vi "Main.vi"() -> ()   [LabVIEW 2019]
uses:
  Code/typeDefs/Parameters.ctl
  Code/typeDefs/MFCIn.ctl
  Code/typeDefs/MFCOut.ctl
  Code/typeDefs/keithleySettings.ctl
  Code/typeDefs/MFCSet.ctl
  <vilib>/Utility/miscctls.llb/LVPointTypeDef.ctl
  <vilib>/DAQmx/read.llb/DAQmx Read (Analog 1D Wfm NChan NSamp).vi
  <vilib>/Analysis/baseanly.llb/Mean (DBL).vi
  <vilib>/DAQmx/write.llb/DAQmx Write (Digital 1D Bool NChan 1Samp 1Line).vi
  <vilib>/DAQmx/write.llb/DAQmx Write (Analog DBL 1Chan 1Samp).vi
  <vilib>/DAQmx/create/channels.llb/DAQmx Create Channel (AO-Voltage-Basic).vi
  <vilib>/DAQmx/miscellaneous.llb/DAQmx Fill In Error Info.vi
  <vilib>/DAQmx/create/channels.llb/DAQmx Create Channel (DO-Digital Output).vi
  <vilib>/DAQmx/create/channels.llb/DAQmx Create Channel (AI-Voltage-Basic).vi
  <vilib>/DAQmx/configure/timing.llb/DAQmx Timing (Sample Clock).vi
  <vilib>/Instr/_visa.llb/VISA Configure Serial Port (Instr).vi
  Code/Scripts/Scripts.lvclass
  Code/SMU/SMU.lvclass
  Code/MFC/MFC.lvclass
  Code/DAQ/DAQ.lvclass
  <resource>/objmgr/daqmx.rc
  <vilib>/Analysis/NI_AALBase.lvlib
  Code/2231A/2231A.lvclass
  <instrlib>/Keithley DMM6500 DAQ6500 Series/Keithley DMM6500 DAQ6500 Series.lvlib
panel:
  out "Visible Resistance":dbl[](array[numeric]) caption="Resistance (Ohms)"
  in  "Names default":string[](array[string])=["Ethanol (%)", "RH (%)", "Temp (C)", "MFC A", "MFC B", "Resistance 1"]
  out "t0 2":dbl
  in  "DevBackgate":bool
  out "Read Time":dbl caption="Read Time (s)"
  out "t0":timestamp
  out "CvsV":T1(graph) caption="Current vs Voltage"
  in  "Timeout Stop":bool
  out "MFC Index":i32
  out "Names":string[](array[string])=["Ethanol (%)", "RH (%)", "Temp (C)", "MFC A", "MFC B", "Resistance 1"]
  in  "Stop":bool
  in  "Tab Control":T2(tab)=enum."Experiment"
  in  "AO_LED":tag="Dev1/ao0"
  in  "DO_Valves":tag="Dev1/port0/line0:1"
  in  "DAQ channels":tag="Dev1/ai0:2"
  in  "Keithley 2450 Sense":refnum<visa-resource-name>="GPIB0::1::INSTR"
  in  "MFC Config":T3={"Tare absP"=FALSE, "Tare Flow"=FALSE, "baud rate (9600)"=19200, "MFC COM Port"="COM5", "Device ID's"=["A", "B"]}
  in  "DAQ Config":T4={"RH/T Sensor VSS (V)"=5.048, "K0"=0.9054, "K1"=-2.995, "Offset"=0.0, "Gain"=1.0, "Samples/Channel/s"=1000.0, "Samples to Average"=1000.0} {"Offset" step=0.01 format="%_3f"; "K1" format="%#_13g"; "K0" format="%#_13g"; "RH/T Sensor VSS (V)" format="%.3g"}
  out "Unprocessed Samples in Queue":u32=5
  out "DPS":dbl=100.0 caption="Data Points / Second"
  in  "Keithley Config":T5={"Source Compliance (A)"=0.1, "Min Voltage (V)"=0.1, "Max Voltage (V)"=3.0, "Source Mode"=0, "Number of Points"=10} {"Number of Points" min=2 step=1; "Source Mode" items=["Voltage", "Current"]; "Min Voltage (V)" min=0.1}
  in  "Keithley wait":sgl caption="Read Delay (s)" min=0 max=100 step=0.25
  in  "DAQ 6510 Switch":refnum<visa-resource-name>="DAQ_6510"
  in  "# of Sensors":dbl=1.0 min=1.0 max=9.0 step=1.0
  in  "Keithley 2450 Source":refnum<visa-resource-name>="GPIB0::2::INSTR"
  in  "Duty Cycle":dbl=0.5 min=0.01 max=0.99 step=0.01
  in  "Freq":dbl=1.0 caption="Freq (Hz)" min=0.1 max=100.0 step=1.0
  in  "Strobe":bool
  in  "Hours to Run":dbl=24.0 min=0.02 max=100.0 step=0.25 format="%#_5g"
  in  "Aquire data":bool
  out "Start Time":timestamp format="%<%I:%M:%S %p>T"
  in  "MFC Set":T6[](array[typedef])=[{"MFC Set"=[{"String"="A", "MFC set"=1000.0}, {"String"="B", "MFC set"=25.0}], "set 1"=FALSE}, {"MFC Set"=[{"String"="A", "MFC set"=1000.0}, {"String"="B", "MFC set"=25.0}], "set 1"=TRUE}] {"MFC Set"."MFC set" step=10.0 format="%.2f"}
  in  "Voltage (V)":dbl(slide) min=0.0 max=10.0 step=0.1 scale=0.0..10.0
  in  "Valves":bool[](array[boolean])=[FALSE, FALSE]
  in  "Plot Data":bool
  out "End Time":timestamp format="%<%I:%M:%S %p>T"
  in  "Save to File":bool
  in  "File Name":string
  out "Current Time (s)":u32
  in  "Aquire data 2":bool
  in  "Test Script":u16(ring) items=["Backgate Test", "Example1", "Example1_rr_bg_40_Nat", "Jaewoo_Test - Copy", "None"]
  out "Script Contents":i32(listbox)
  in  "Sensors":bool[](array[boolean])=[TRUE, FALSE, FALSE, FALSE, FALSE, FALSE, FALSE, FALSE, FALSE]
  out "Backgate Display":cluster{"all rows":dbl[], "all rows":dbl[]}(graph)
  in  "Increment (V)":dbl=1.0 min=0.0 max=63.0
  in  "Range (V)":dbl=60.0 min=1.0 max=60.0
  in  "Backgate":bool
  in  "Style":u16(ring) items=["Ramp+-", "Pos-Neg", "Ramp", "0 Ramp", "Double+-"]
  out "BG Time (s)":dbl
  out "Computer Read Time (s)":dbl
  out "Keithley 2450 Source":errorcluster
  out "LED_AO":errorcluster
  out "3-Valve_DO":errorcluster
  out "DAQ_IO (RH,Temp,Eth)":errorcluster
  out "MFC_IO":errorcluster
  out "Keithley 2450 Sense":errorcluster
  out "DAQ 6510 Switch":errorcluster
  out "Resistance Proper":dbl[][](array[numeric]) caption="Resistance"
  in  "Clear DAQ":bool
  out "MFCArray":T7[](array[typedef])=[{"Gas"="", "Setpoint"=0.0, "MassFlow"=0.0, "T ºC"=0.0, "P(PSI)"=0.0, "ID"="-"}, {"Gas"="", "Setpoint"=0.0, "MassFlow"=0.0, "T ºC"=0.0, "P(PSI)"=0.0, "ID"="-"}] {"MassFlow" format="%.2f"; "Setpoint" format="%.2f"}
  out "Waveform Chart":waveform(dbl)[](graph)=[{"t0"=timestamp(3675342615.977705 s since 1904-01-01), "dt"=0.01, "Y"=[0.0007680409200236937]}, {"t0"=timestamp(3675342615.977705 s since 1904-01-01), "dt"=0.01, "Y"=[0.0105205510693704]}, {"t0"=timestamp(3675342615.977705 s since 1904-01-01), "dt"=0.01, "Y"=[89.00820200660893]}, {"t0"=timestamp(3675342615.977705 s since 1904-01-01), "dt"=0.01, "Y"=[117.62674839380017]}, {"t0"=timestamp(3675342615.977705 s since 1904-01-01), "dt"=0.01, "Y"=[0.0]}, {"t0"=timestamp(3675342615.977705 s since 1904-01-01), "dt"=0.01, "Y"=[0.0]}]
  out "T":dbl caption="T  (ºC)" format="%.2g"
  out "RH":dbl caption="RH  (%)" format="%.2g"
  out "Eth":dbl caption="Ethanol (%)" format="%.3g"
  # "Created By Lukas Scarfe\nEngineering Physics"
  # "Save to File"
  # "LED"
  # "1"
  # "2"
  # "Backgate Configuration"
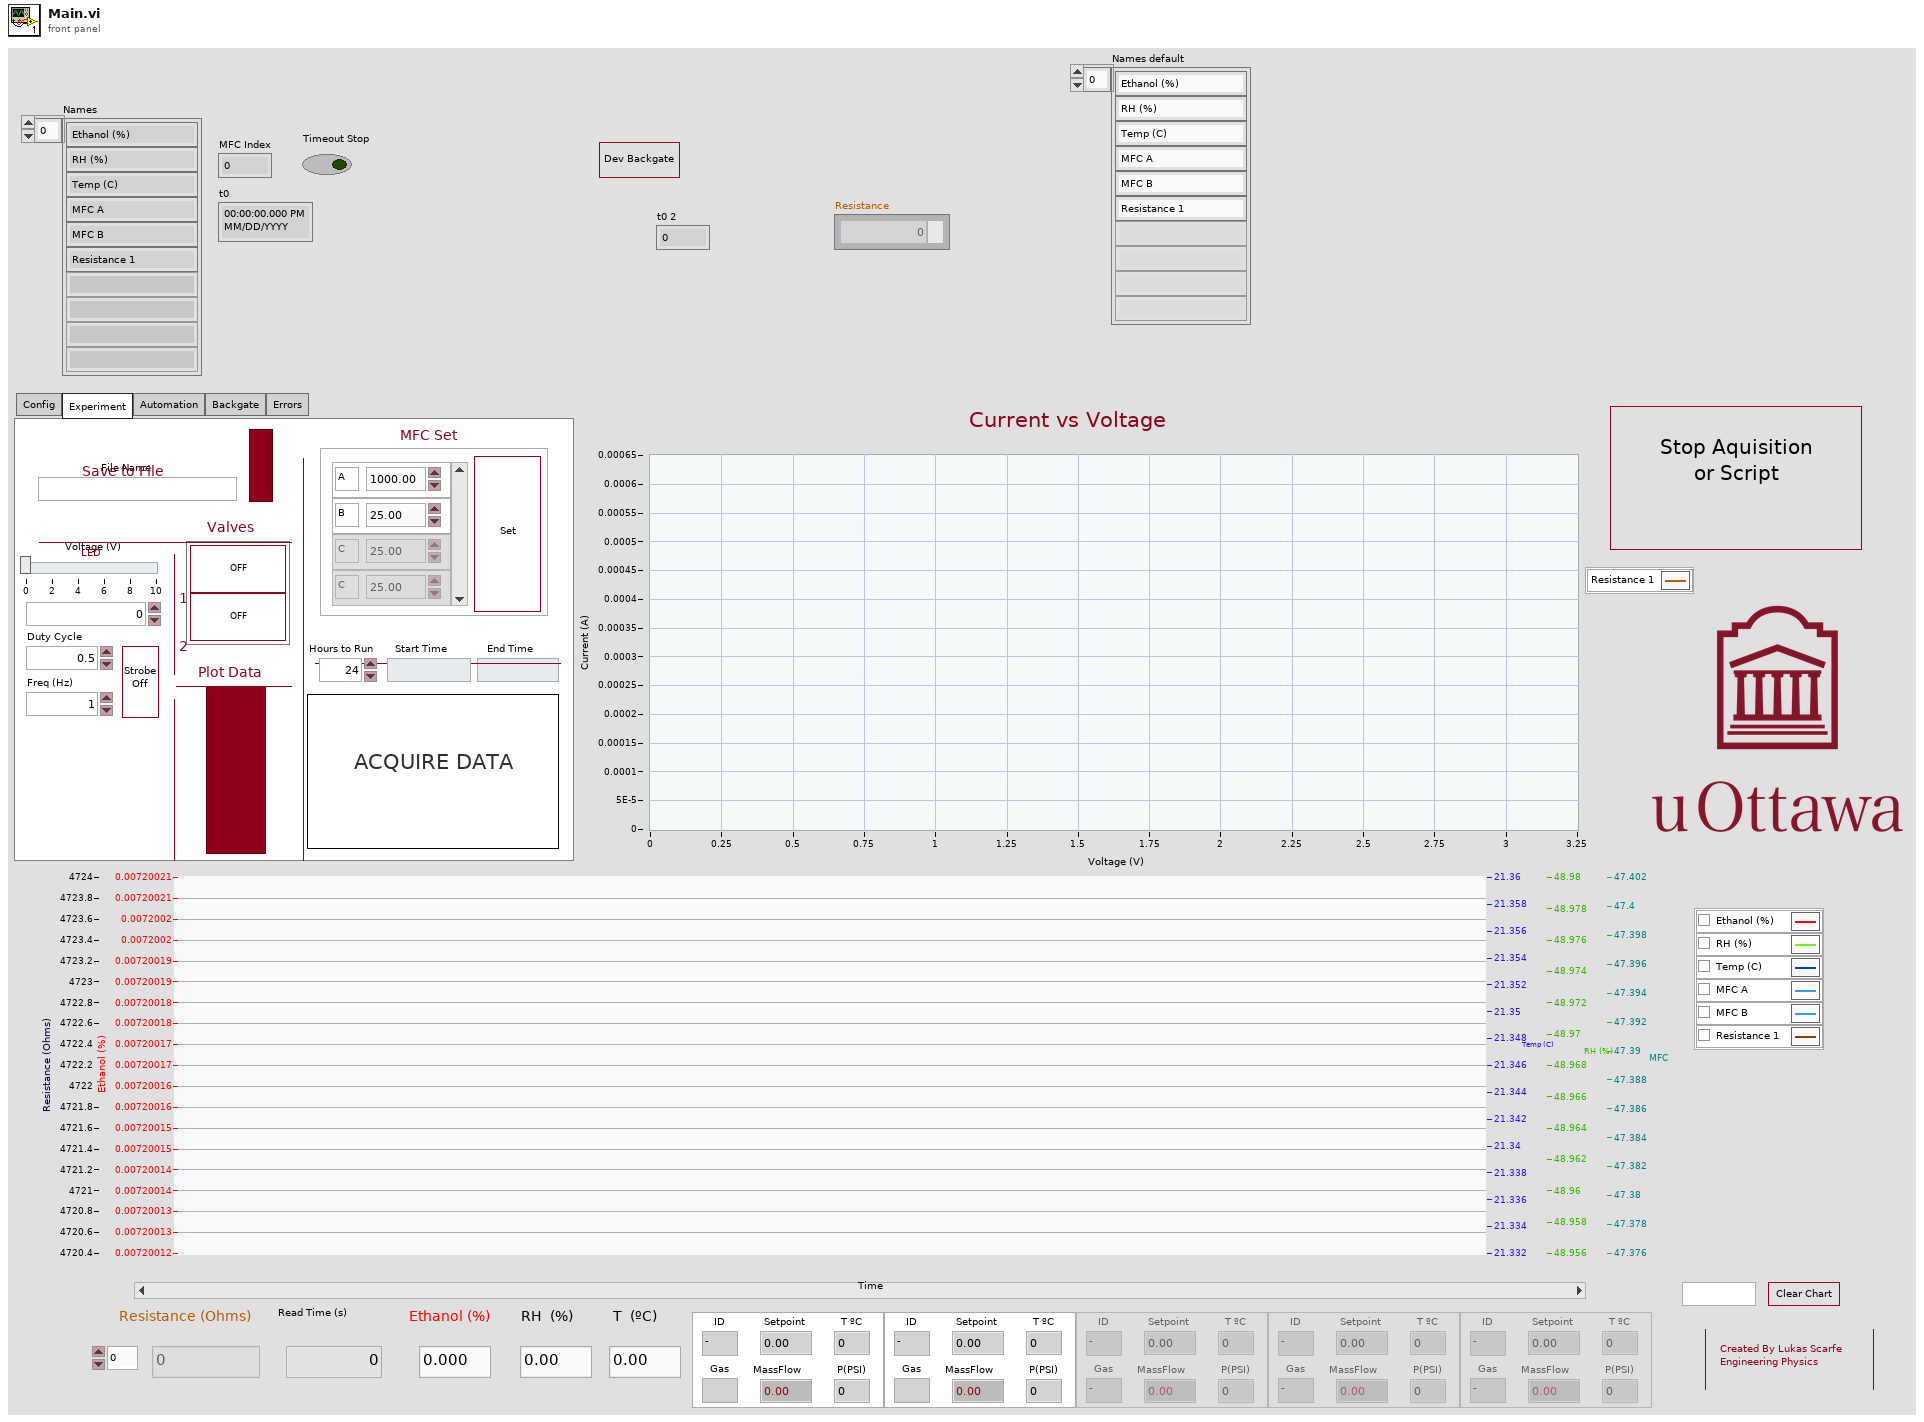
[diagram p1: front panel]
types:
  T1 = cluster{"All Values Out":sgl[], "All Values Out":sgl[]}[]
  T2 = enum32{"Config", "Experiment", "Automation", "Backgate", "Errors"}
  T3 = typedef "MFCIn.ctl" = cluster{"Tare absP":bool, "Tare Flow":bool, "baud rate (9600)":u32, "MFC COM Port":refnum<visa-resource-name>, "Device ID's":string[]}
  T4 = typedef "Parameters.ctl" = cluster{"RH/T Sensor VSS (V)":dbl, "K0":dbl, "K1":dbl, "Offset":dbl, "Gain":dbl, "Samples/Channel/s":dbl, "Samples to Average":dbl}
  T5 = typedef "keithleySettings.ctl" = cluster{"Source Compliance (A)":dbl, "Min Voltage (V)":dbl, "Max Voltage (V)":dbl, "Source Mode":u16, "Number of Points":u32}
  T6 = typedef "MFCSet.ctl" = cluster{"MFC Set":cluster{"String":string, "MFC set":dbl}[], "set 1":bool}
  T7 = typedef "MFCOut.ctl" = cluster{"Gas":string, "Setpoint":dbl, "MassFlow":dbl, "T ºC":dbl, "P(PSI)":dbl, "ID":string}
  T8 = enum32{"invalid app kind", "Development System", "Run Time System", "Student Edition", "Embedded LabVIEW", "Evaluation", "Custom"}
  T9 = typedef "LVPointTypeDef.ctl" = cluster{"Horizontal":i16, "Vertical":i16}
  T10 = cluster{"array":sgl[], "Best Linear Fit":dbl[]}[]
  T11 = enum8{"Enabled", "Disabled", "Disabled and Grayed Out"}
  T12 = cluster{"All Values Out":sgl[], "All Values Out":sgl[]}
  T13 = cluster{"MFC Set":cluster{"String":bool, "MFC set":bool}[], "set 1":bool}
  T14 = typedef "Graph.ctl" = cluster{"Ethanol":dbl, "RH":dbl, "Temp":dbl, "MFC A":dbl, "MFC B":dbl, "Resistances":dbl[][]}
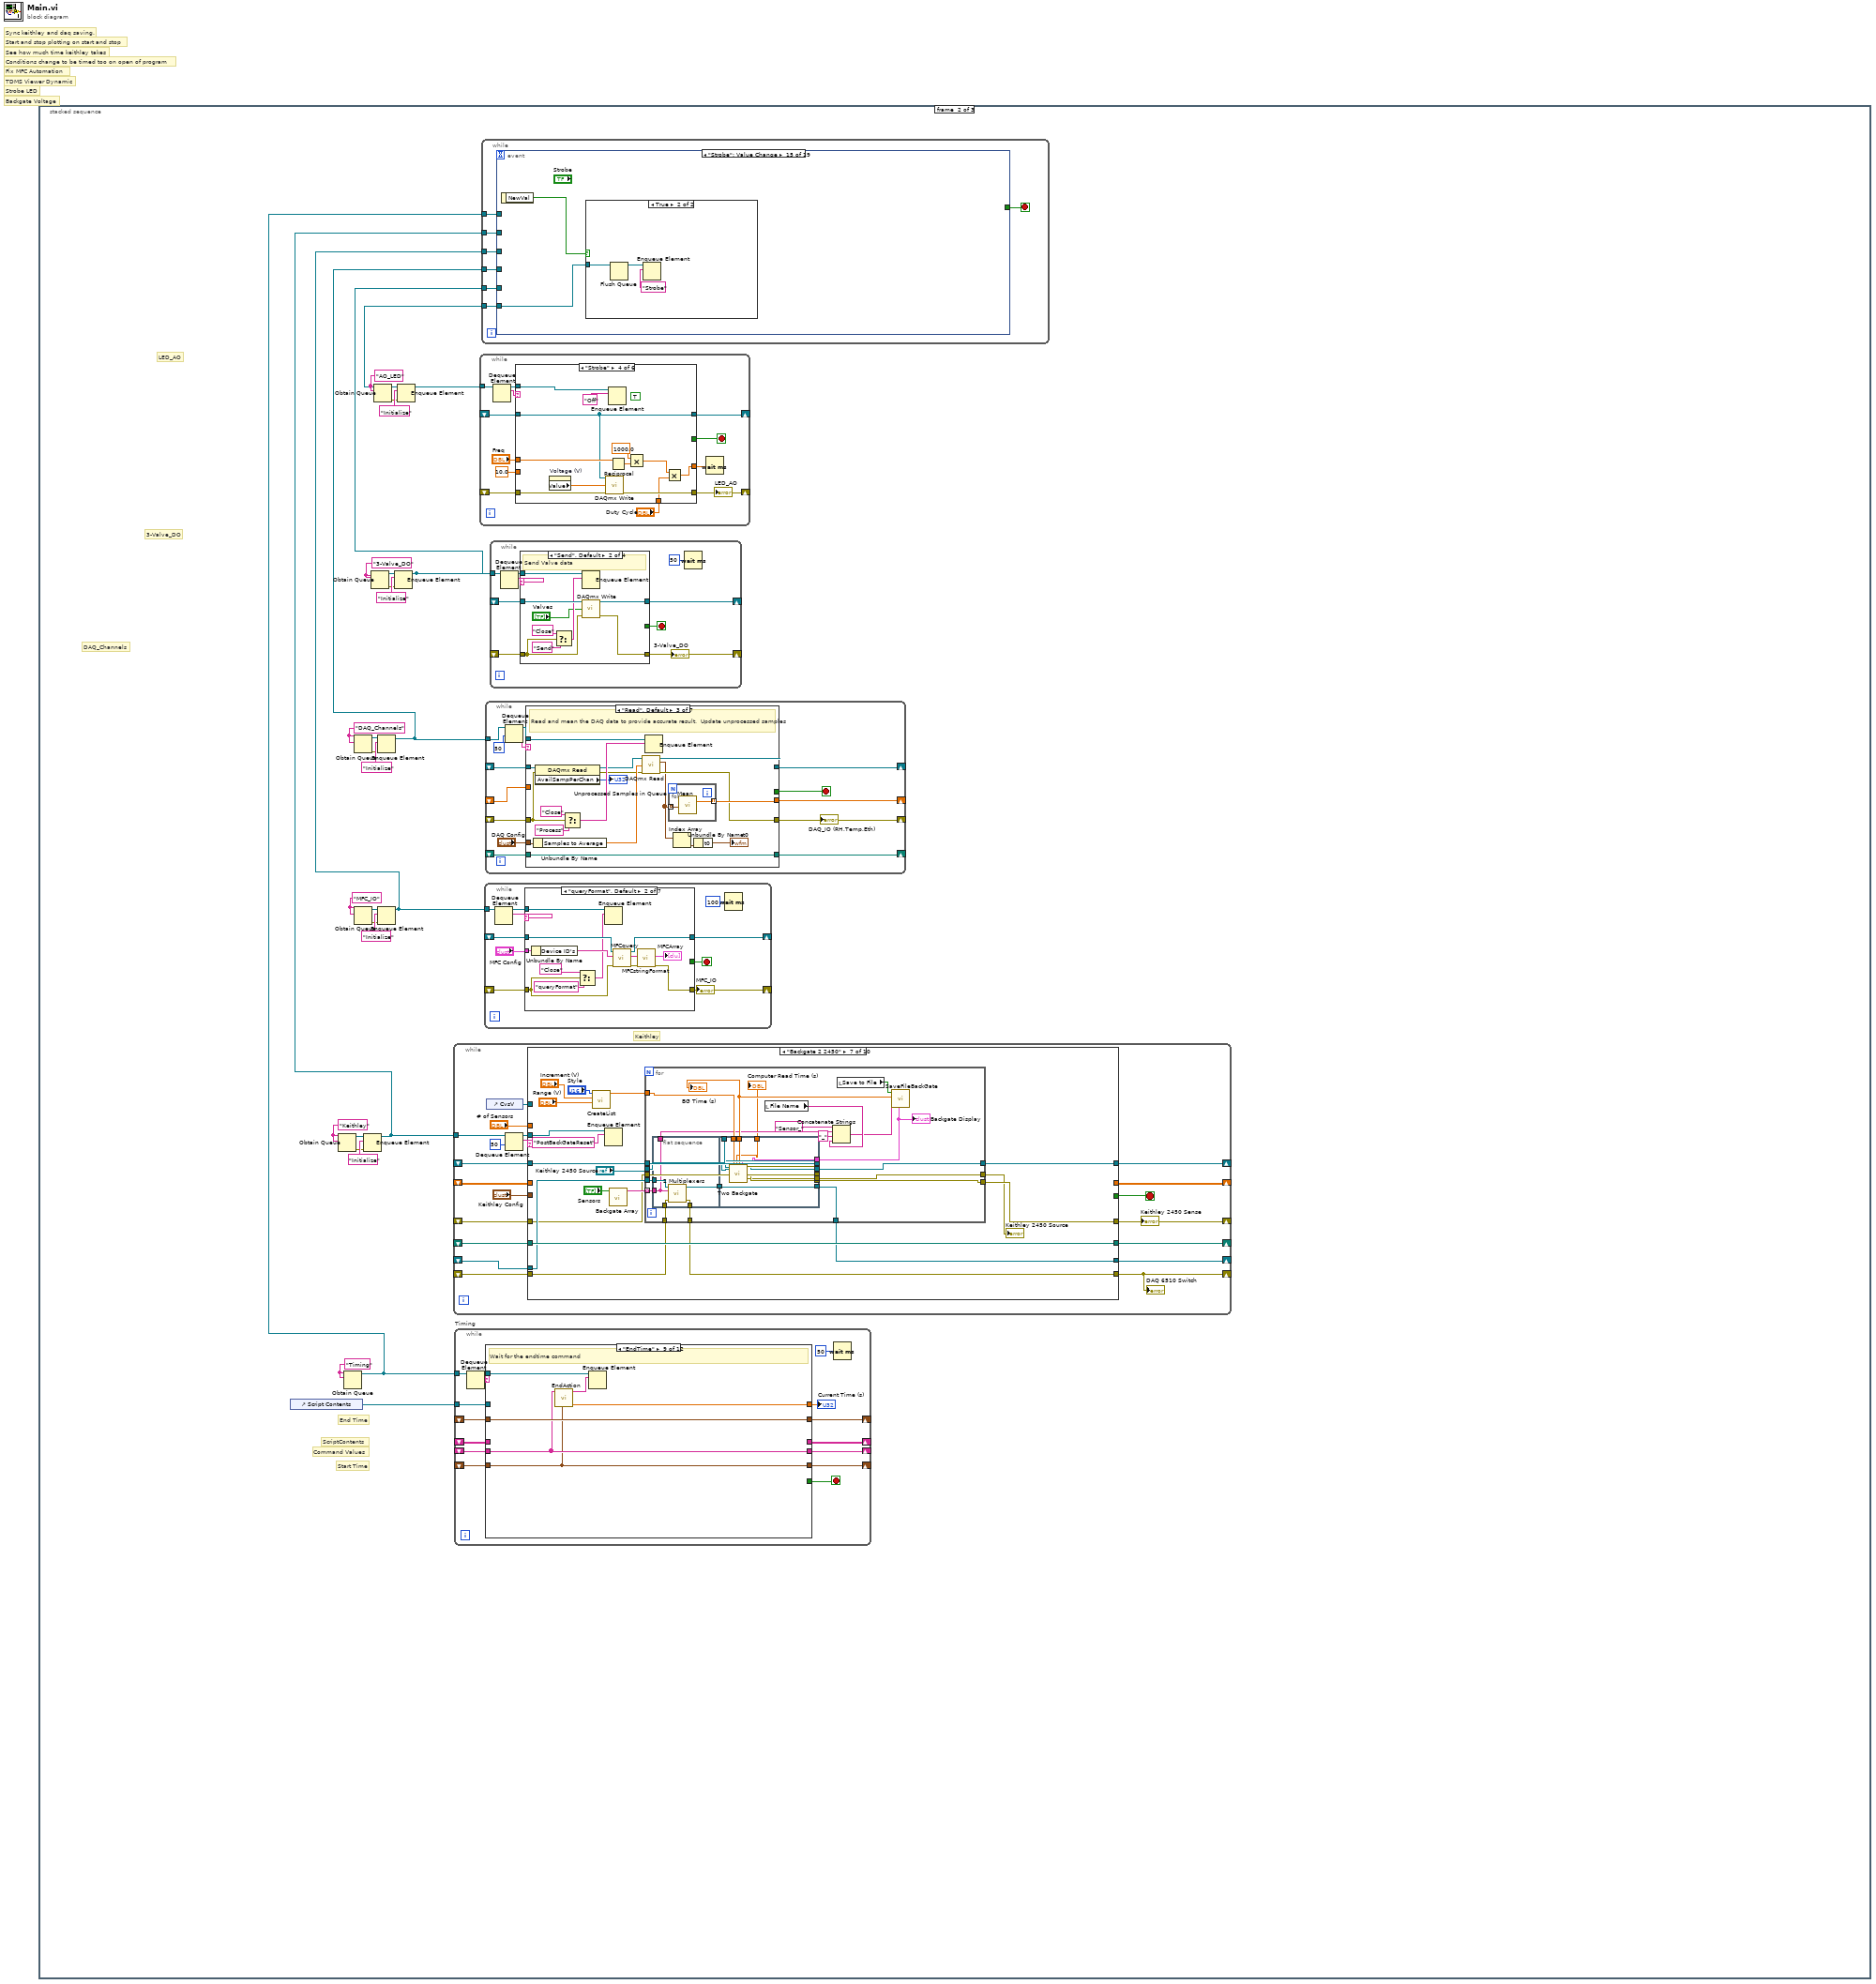
[diagram p0: block diagram]
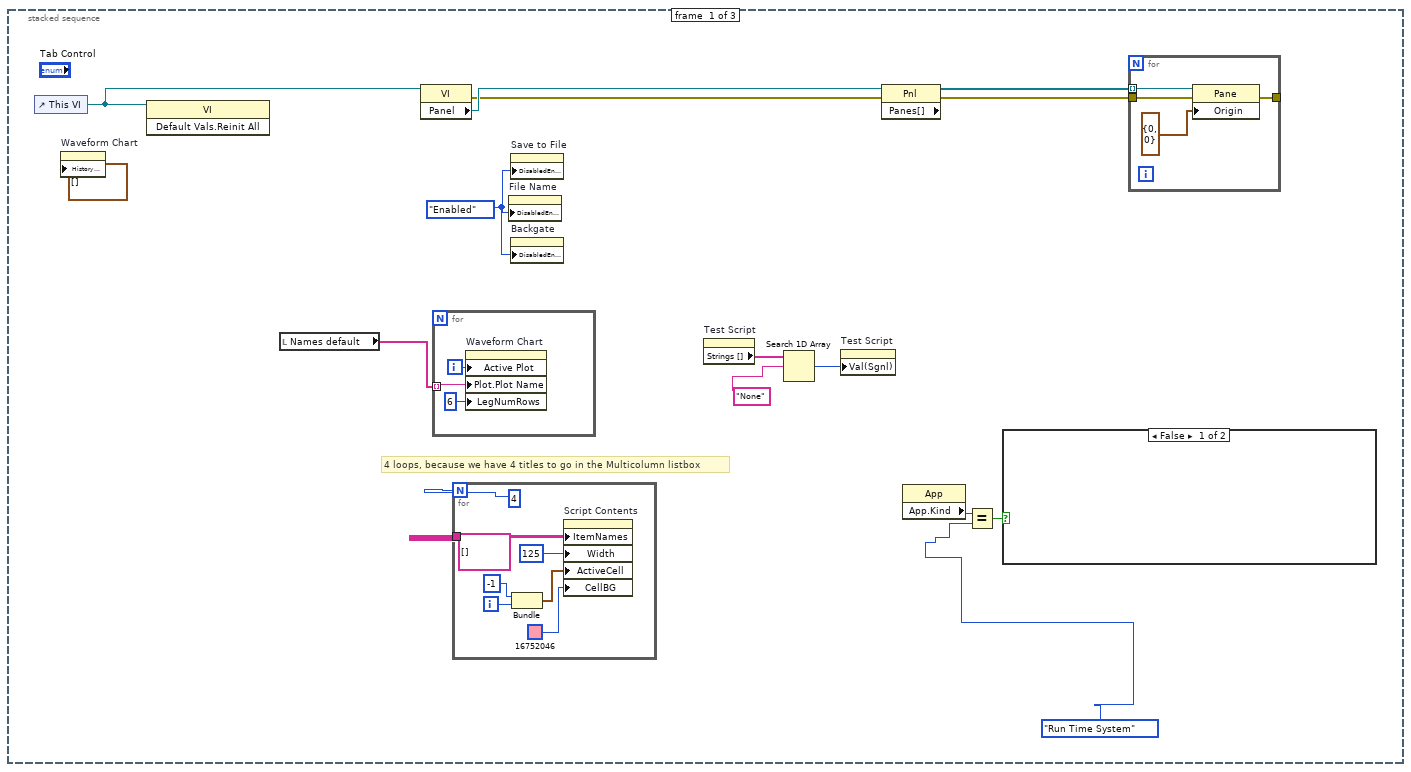
[diagram p2: hidden frame]
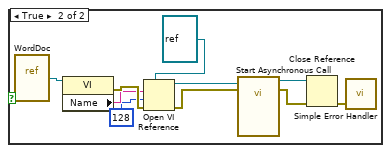
[diagram p3: hidden frame]
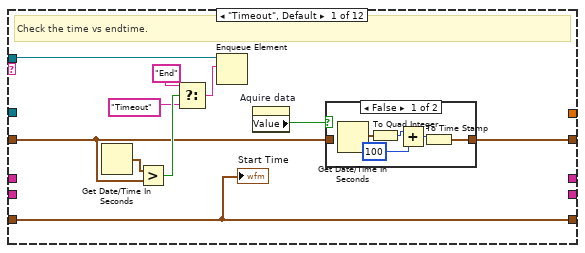
[diagram p4: hidden frame]
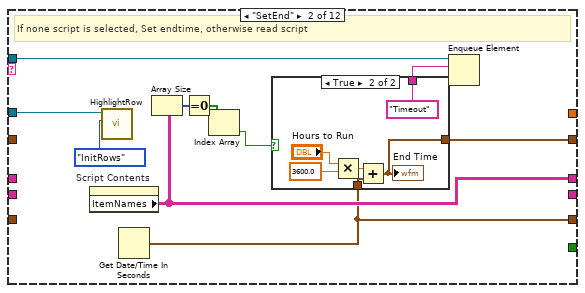
[diagram p6: hidden frame]
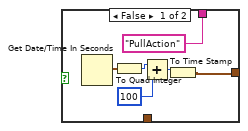
[diagram p7: hidden frame]
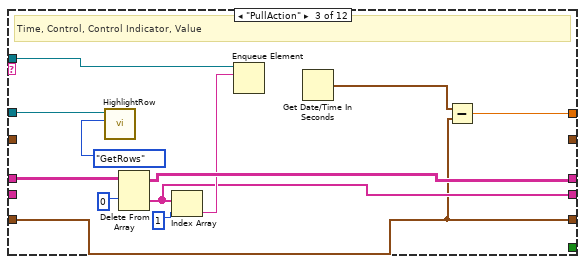
[diagram p8: hidden frame]
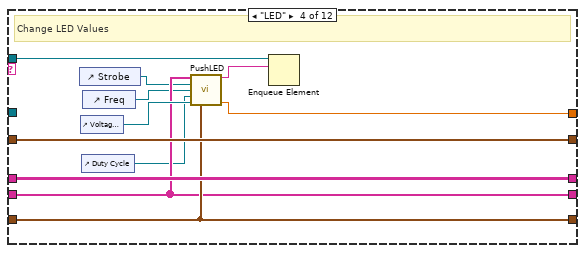
[diagram p9: hidden frame]
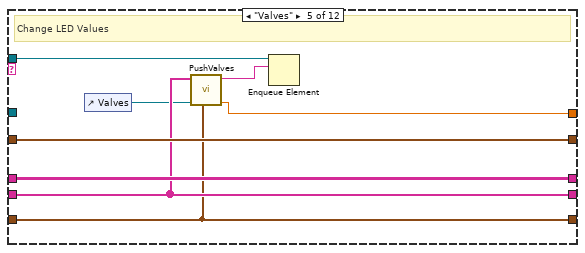
[diagram p10: hidden frame]
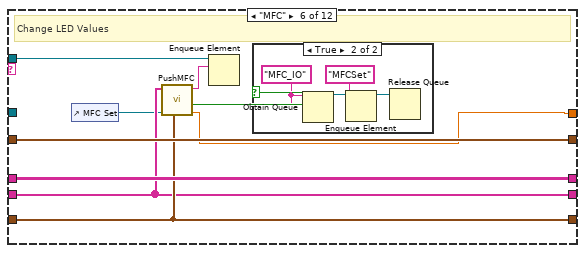
[diagram p11: hidden frame]
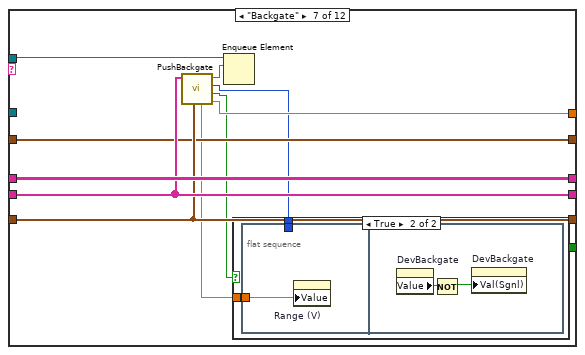
[diagram p13: hidden frame]
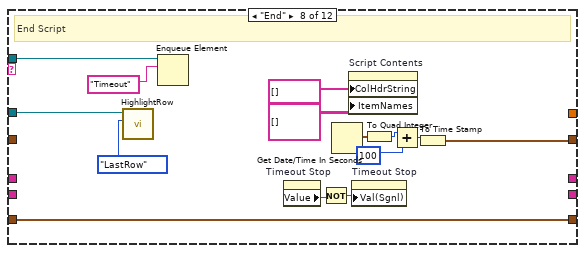
[diagram p15: hidden frame]
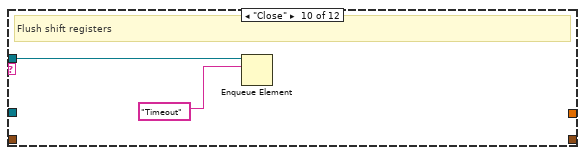
[diagram p16: hidden frame]
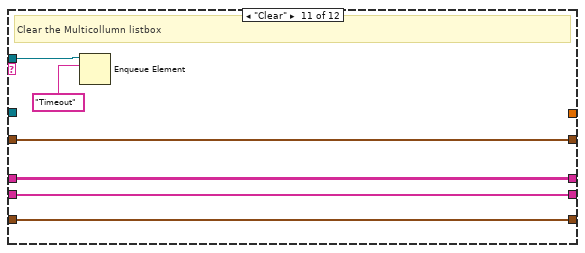
[diagram p17: hidden frame]
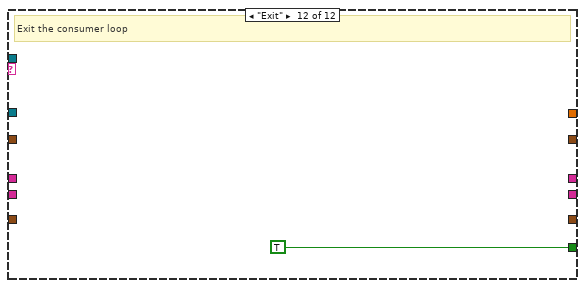
[diagram p18: hidden frame]
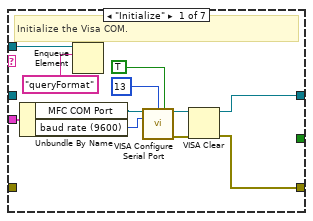
[diagram p19: hidden frame]
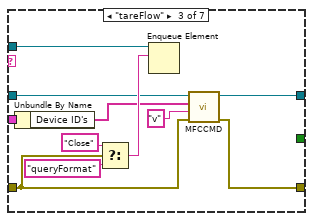
[diagram p20: hidden frame]
diagram:
  # "Start and stop plotting on start and stop"
  # "Conditions change to be timed too on open of program"
  # "Sync keithley and daq saving."
  # "See how much time keithley takes"
  # "Fix MFC Automation"
  # "TDMS Viewer Dynamic"
  # "Backgate Voltage"
  # "Strobe LED"
  n1 = stacked-sequence {
    frame #0 {
      w1 = T11."Enabled" ("Disabled")
      # "4 loops, because we have 4 titles to go in the Multicolumn listbox"
      n2 = control-ref of="This VI"() -> (w11:refnum<vi>)
      n3 = property on="Waveform Chart" class="WFChart (strict)"("History Data"=waveform(dbl)[][] []) -> ()  [unwired: 2 in, 2 out]
      n4 = invoke class="VI" method="Default Vals.Reinit All"(reference=w11) -> ()  [unwired: 2 in, 3 out]
      n5 = local read "Names default"() -> (w2:string[])
      n6 = property class="VI"(reference=w11) -> (error out=w14:errorcluster, "Panel"=w15:refnum<vi>)  [unwired: 1 in, 1 out]
      n7 = for {
        tunnel: w2 -> [w38] mode=indexing
        i -> [w39]
        n8 = property on="Waveform Chart" class="WFChart (strict)"("Active Plot"=w39, "Plot.Plot Name"=w38, "LegNumRows"=u32 6 ("Legend:Number of Rows")) -> ()  [unwired: 2 in, 2 out]
      }
      n9 = for {
        N: 4 -> [_]
        tunnel: string[][] [] ("Item Names") -> [w32]
        i -> [w30]
        n10 = Bundle(-1, w30) -> (w29:cluster{i32, i32})  [unwired: 1 in]
        n11 = property on="Script Contents" class="MCListbox (strict)"("ItemNames"=w32, "Width"=u32 125 ("Size:Width"), "ActiveCell"=w29, "CellBG"=u32 16752046) -> ()  [unwired: 2 in, 2 out]
      }
      n12 = property on="File Name" class="Str"("DisabledEnum"=w1) -> ()  [unwired: 2 in, 2 out]
      n13 = property on="Save to File" class="Bool (strict)"("DisabledEnum"=w1) -> ()  [unwired: 2 in, 2 out]
      n14 = property on="Backgate" class="Bool"("DisabledEnum"=w1) -> ()  [unwired: 2 in, 2 out]
      n15 = property on="Test Script" class="Ring (strict)"() -> ("Strings []"=w7:string[])  [unwired: 2 in, 2 out]
      n16 = Search 1D Array(1D array=w7, element="None") -> (index of element=w6:i32)  [unwired: 1 in]
      n17 = property on="Test Script" class="Ring (strict)"("Val(Sgnl)"=w6) -> ()  [unwired: 2 in, 2 out]
      n18 = property class="Pnl"(reference=w15, error in=w14) -> (error out=w12:errorcluster, "Panes[]"=w13:refnum<vi>[])  [unwired: 1 out]
      n19 = property class="App"() -> ("App.Kind"=w4:T8)  [unwired: 2 in, 2 out]
      n20 = Equal?(x=w4, y=T8."Run Time System" ("Application:Kind")) -> (x = y?=w5:bool)
      n21 = case shown="False" w5 {
        frame False {
        }
        frame True {
          n22 = vi-ref "WordDoc.vi"() -> (w19:refnum<vi>)
          n23 = property class="VI"(reference=w19) -> (error out=w21:errorcluster, "Name"=w20:string)  [unwired: 1 in, 1 out]
          n24 = Open VI Reference(type specifier VI Refnum (for type only)=refnum<vi> refnum, vi path=w20, options=128, error in (no error)=w21) -> (vi reference=w22:refnum<vi>, error out=w24:errorcluster)  [unwired: 2 in]
          n25 = call-by-ref "Start Asynchronous Call"(reference=w22, error in=w24) -> (reference out=w23:refnum<vi>, error out=w25:errorcluster)  [unwired: 11 in, 1 out]
          n26 = Close Reference(reference=w23, error in (no error)=w25) -> (error out=w26:errorcluster)
          n27 = call <vilib>:"Simple Error Handler.vi"("error in (no error)"=w26) -> ()  [unwired: 4 in, 5 out]
        }
      }
      n28 = for {
        tunnel: w13 -> [w36] mode=indexing
        tunnel: w12 -> [w35]
        tunnel: [w33] -> _
        n29 = property class="Pane"(reference=w36, error in=w35, "Origin"=T9 {"Horizontal"=0, "Vertical"=0}) -> (error out=w33:errorcluster)  [unwired: 1 out]
      }
    }
    frame #1 {
      w43 = "MFC_IO" ("name (unnamed)")
      w46 = "DAQ_Channels" ("name (unnamed)")
      w44 = "3-Valve_DO" ("name (unnamed)")
      w54 = "AO_LED" ("name (unnamed)")
      w59 = "Keithley" ("name (unnamed)")
      w62 = "Timing" ("name (unnamed)")
      # "Keithley"
      # "3-Valve_DO"
      # "LED_AO"
      # "DAQ_Channels"
      # "Command Values"
      # "ScriptContents"
      # "Start Time"
      # "End Time"
      n30 = control-ref of="Script Contents"() -> (w60:refnum<vi>)
      n31 = Obtain Queue(name (unnamed)=w59, element data type=w59) -> (queue out=w57:refnum<queue>, error out=w56:errorcluster)  [unwired: 3 in, 1 out]
      n32 = Obtain Queue(name (unnamed)=w62, element data type=w62) -> (queue out=w61:refnum<queue>)  [unwired: 3 in, 2 out]
      n33 = Obtain Queue(name (unnamed)=w43, element data type=w43) -> (queue out=w41:refnum<queue>, error out=w42:errorcluster)  [unwired: 3 in, 1 out]
      n34 = Obtain Queue(name (unnamed)=w46, element data type=w46) -> (queue out=w40:refnum<queue>, error out=w45:errorcluster)  [unwired: 3 in, 1 out]
      n35 = Enqueue Element(queue=w57, element="Initialize", error in (no error)=w56) -> (queue out=w63:refnum<queue>)  [unwired: 1 in, 2 out]
      n36 = Obtain Queue(name (unnamed)=w44, element data type=w44) -> (queue out=w48:refnum<queue>, error out=w49:errorcluster)  [unwired: 3 in, 1 out]
      n37 = Obtain Queue(name (unnamed)=w54, element data type=w54) -> (queue out=w52:refnum<queue>, error out=w53:errorcluster)  [unwired: 3 in, 1 out]
      n38 = Enqueue Element(queue=w41, element="Initialize", error in (no error)=w42) -> (queue out=w67:refnum<queue>)  [unwired: 1 in, 2 out]
      n39 = Enqueue Element(queue=w40, element="Initialize", error in (no error)=w45) -> (queue out=w66:refnum<queue>)  [unwired: 1 in, 2 out]
      n40 = Enqueue Element(queue=w48, element="Initialize", error in (no error)=w49) -> (queue out=w64:refnum<queue>)  [unwired: 1 in, 2 out]
      n41 = Enqueue Element(queue=w52, element="Initialize", error in (no error)=w53) -> (queue out=w65:refnum<queue>)  [unwired: 1 in, 2 out]
      n42 = while {
        shift-right: [w521] -> _
        shift-left: _ -> [w525]
        shift-right: [w524] -> _
        shift-left: _ -> [w523]
        tunnel: w63 -> [w522]
        shift-right: [w519] -> _
        shift-left: _ -> [w518]
        shift-right: [w517] -> _
        shift-left: _ -> [w516]
        shift-right: [w513] -> _
        shift-left: _ -> [w511]
        shift-right: [w512] -> _
        shift-left: _ -> [w510]
        stop <- w520 stop-if-true
        n43 = control-ref of="CvsV"() -> (w514:refnum<vi>)
        n44 = Dequeue Element(queue=w522, timeout in ms (-1)=50) -> (queue out=w527:refnum<queue>, element=w526:string)  [unwired: 1 in, 2 out]
        n45 = case shown="\"Backgate 2 2450\"" w526 {
          tunnel: w527 -> [w549 w554 w578 w602 w608 w627 w645 w692 w705 _]
          tunnel: [_ _ _ _ _ _ _ _ _ TRUE] -> w520
          tunnel: [w535 w552 _ w599 w619 w623 w638 w694 w708 w716] -> w521
          tunnel: w525 -> [_ w552 w571 w599 w619 w623 w629 w695 w710 w715]
          tunnel: [w536 w556 w568 w600 w614 w624 w639 w697 w707 _] -> w524
          tunnel: w523 -> [_ w556 w569 w600 w614 w624 w640 w698 w709 w717]
          tunnel: [_ _ w564 _ w613 _ _ w688 _ _] -> w519
          tunnel: w518 -> [_ _ _ w594 w613 _ _ w688 _ _]
          tunnel: [_ w555 w574 w592 w615 w628 w647 w691 _ _] -> w517
          tunnel: w516 -> [_ _ w574 w593 w615 w628 w647 w691 _ _]
          tunnel: "Keithley Config" -> [w538 _ w566 w590 _ _ _ w696 _ _]
          tunnel: w514 -> [w540 _ _ _ _ _ _ _ _ _]
          tunnel: [w531 w551 w567 w597 w606 w621 w630 w690 w700 _] -> w513
          tunnel: [w530 w550 w572 w596 w605 w620 w631 w689 w701 w712] -> w512
          tunnel: w511 -> [_ w551 w570 w597 w606 w621 w641 w690 w700 w714]
          tunnel: w510 -> [_ w550 w572 w596 w605 w620 w634 w689 w702 w713]
          tunnel: "# of Sensors" -> [w528 _ w562 _ _ _ _ _ _ _]
          frame "Initialize" {
            w542 = u16 0 items=["Init", "Increment"] ("Ring")
            # "Initialize the Keithley"
            n46 = local read "Save to File"() -> (w545:bool)
            n47 = call "BackgateRead.vi"("GrphChrt Refnum"=w540, "Ring"=w542) -> ()  [unwired: 5 in, 5 out]
            n48 = Select(t="File", s=w545, f="Read" ("element")) -> (s? t:f=w546:string)
            n49 = property on="CvsV" class="XYGraph (strict)"("Value"=T10 [] ("CvsV"), "XScale.NameLbl.Text"="Voltage (V)" ("Y Scale.Name Label.Text"), "YScale.NameLbl.Text"="Current (A)" ("X Scale.Name Label.Text"), "Caption.Text"="Current vs Voltage", "LegNumRows"=w528) -> ()  [unwired: 2 in, 2 out]
            n50 = Enqueue Element(queue=w549, element=w546) -> ()  [unwired: 2 in, 3 out]
            n51 = call <vilib>:"High Resolution Relative Seconds.vi"() -> ("relative seconds"=w534:dbl)
            n52 = property on="t0 2" class="DigNum (strict)"("Value"=w534) -> ()  [unwired: 2 in, 2 out]
            n53 = call "SMU2450Init.vi"("Keithley Config"=w538, "Keithley 2400 Name"="Keithley 2450 Sense") -> ("error out"=w535:errorcluster, "VISA resource name out"=w536:refnum<visa-resource-name>)  [unwired: 8 in]
            n54 = call <instrlib>:"Initialize.vi"("VISA resource name"="DAQ 6510 Switch") -> ("error out"=w533:errorcluster, "VISA resource name out"=w532:refnum<visa-resource-name>)  [unwired: 9 in]
            n55 = call <instrlib>:"Open All Channels.vi"("error in (no error)"=w533, "VISA resource name"=w532) -> ("error out"=w530:errorcluster, "VISA resource name out"=w531:refnum<visa-resource-name>)  [unwired: 8 in]
          }
          frame "File" {
            # "Create desired file"
            n56 = case shown="No Error" w552 {
              tunnel: [w558 _] -> w555
              frame No Error {
                n57 = local read "File Name"() -> (w557:string)
                n58 = call "CreateFileIVPath.vi"("DAQ File Name"=w557) -> ("appended path 2"=w558:path)  [unwired: 9 in, 1 out]
              }
              frame Error {
              }
            }
            n59 = Enqueue Element(queue=w554, element="Read") -> ()  [unwired: 2 in, 3 out]
          }
          frame "Read", Default {
            # "Read data from the keithley"
            n60 = local read "t0 2"() -> (w573:dbl)
            n61 = call "Multiread.vi"("Keithley 2450"=w569, "Keithley Config"=w566, "6510"=w570, "Number of Sensors"=w562, "2450 error in"=w571, "6510 error in"=w572, "t0 2"=w573) -> ("2450 Visa"=w568:refnum<visa-resource-name>, "6510 Visa"=w567:refnum<visa-resource-name>, "All Values Out"=w564:sgl[][][], "Resistance (ohm) Out"=w560:dbl[][], "Total Read Time"=→"Read Time":dbl)  [unwired: 4 in]
            "Resistance Proper" <- w560
            n62 = Select(t="Close" ("element"), s=w571, f="Process" ("element")) -> (s? t:f=w576:string)
            n63 = Enqueue Element(queue=w578, element=w576) -> ()  [unwired: 2 in, 3 out]
            n64 = local read "Plot Data"() -> (w563:bool)
            n65 = for {
              tunnel: w560 -> [w581] mode=indexing
              tunnel: [w579] -> w559 mode=indexing
              n66 = Index Array(array=w581, index=2) -> (element=w579:dbl)
            }
            "Visible Resistance" <- w559
            n67 = case shown="True" w563 {
              tunnel: [_ w584] -> w565
              tunnel: w562 -> [_ w583]
              tunnel: w564 -> [_ w582]
              frame False {
              }
              frame True {
                n68 = for {
                  N: w583 -> [_]
                  tunnel: [w585] -> w584 mode=indexing
                  tunnel: w582 -> [w586] mode=indexing
                  n69 = Index Array(array=w586) -> (element #1=w588:sgl[], element #2=w587:sgl[])  [unwired: 4 in]
                  n70 = Bundle("All Values Out"=w588, "All Values Out"=w587) -> (w585:T12)  [unwired: 1 in]
                }
              }
            }
            "CvsV" <- w565
          }
          frame "Process" {
            # "Process the data aquired. Initialize wait timer"
            n71 = Unbundle By Name(w590) -> ("Number of Points"=w589:u32)
            n72 = Select(t="Close" ("element"), s=w599, f="CheckTime" ("element")) -> (s? t:f=w601:string)
            n73 = Enqueue Element(queue=w602, element=w601) -> ()  [unwired: 2 in, 3 out]
            n74 = local read "# of Sensors"() -> (w591:dbl)
            n75 = call "Timer.vi"("State"=enum16{"GetTime", "InitTime"}."InitTime") -> ()  [unwired: 10 in, 1 out]
            n76 = local read "Aquire data"() -> (w595:bool)
            n77 = call "MultiFileDocument.vi"("Number of points"=w589, "Number of sensors"=w591, "Aquire Data"=w595, "Multivalues"=w594, "File Path In"=w593) -> ("file path out"=w592:path)  [unwired: 6 in]
          }
          frame "CheckTime" {
            # "Check timer time vs wait time"
            n78 = call "Timer.vi"("State"=enum16{"GetTime", "InitTime"}."GetTime") -> ("Timer (s)"=w617:dbl)  [unwired: 10 in]
            n79 = Greater?(x=w617, y="Keithley wait") -> (0:w612:bool)
            n80 = Select(t="Read", s=w612, f="CheckTime") -> (s? t:f=w609:string)
            n81 = Enqueue Element(queue=w608, element=w609) -> ()  [unwired: 2 in, 3 out]
            n82 = Wait (ms)(milliseconds to wait=u32 50) -> ()  [unwired: 1 out]
          }
          frame "ResetTimestamp" {
            n83 = Wait (ms)(milliseconds to wait=u32 100) -> ()  [unwired: 1 out]
            n84 = Enqueue Element(queue=w627, element="Read") -> ()  [unwired: 2 in, 3 out]
            n85 = call <vilib>:"High Resolution Relative Seconds.vi"() -> ("relative seconds"=→"t0 2":dbl)
          }
          frame "Backgate 2 2450" {
            n86 = call "CreateList.vi"("Range"="Range (V)", "Increment (V)"="Increment (V)", "Style"="Style") -> ("Ramp Pattern"=w635:dbl[])  [unwired: 8 in]
            n87 = Enqueue Element(queue=w645, element="PostBackGateReset") -> ()  [unwired: 2 in, 3 out]
            n88 = call "Backgate Array.vi"("Sensors"="Sensors") -> ("Array"=w632:string[])  [unwired: 10 in]
            n89 = for {
              tunnel: w641 -> [w668]
              tunnel: w640 -> [w662]
              tunnel: [w656] -> w639
              tunnel: [w655] -> w638
              tunnel: [w654] -> w637
              tunnel: "Keithley 2450 Source" -> [w661]
              tunnel: w635 -> [w659]
              tunnel: w634 -> [w667]
              tunnel: w632 -> [w666] mode=indexing
              tunnel: [w665] -> w631
              tunnel: [w664] -> w630
              tunnel: w629 -> [w660]
              n90 = flat-sequence {
                tunnel: w668 -> [w674]
                tunnel: w667 -> [w673]
                tunnel: w666 -> [w670]
                tunnel: [w672] -> w665
                tunnel: [w671] -> w663
                tunnel: [w670] -> w653
                tunnel: [w685] -> w664
                tunnel: w663 -> [w685]
                tunnel: w662 -> [w684]
                tunnel: w661 -> [w683]
                tunnel: w660 -> [w682]
                tunnel: w659 -> [w681]
                tunnel: [w680] -> w658
                tunnel: [w679] -> w657
                tunnel: [w678] -> w656
                tunnel: [w677] -> w655
                tunnel: [w676] -> w654
                tunnel: [w675] -> w648
                frame #0 {
                  n91 = call "2 Multiplexers.vi"("6510 Error In"=w673, "String"=w670, "6510 In"=w674) -> ("6510 Error Out"=w672:errorcluster, "6510 Out"=w671:refnum<visa-resource-name>)  [unwired: 7 in]
                }
                frame #1 {
                  n92 = call "Two Backgate.vi"("Sense"=w684, "Source"=w683, "Sense error in"=w682, "Input sweep"=w681) -> ("Read Time"=w675:dbl, "BG Time Taken (s)"=w680:dbl, "XY Graph"=w679:cluster{dbl[], "Ramp Pattern":dbl[]}, "Sense Out"=w678:refnum<visa-resource-name>, "Sense error out"=w677:errorcluster, "Source error out"=w676:errorcluster)  [unwired: 7 in, 3 out]
                }
              }
              n93 = local read "File Name"() -> (w651:string)
              n94 = Concatenate Strings("Sensor_" ("string"), w653, "_" ("string"), w651) -> (w649:string)
              n95 = local read "Save to File"() -> (w669:bool)
              n96 = call "SaveFileBackGate.vi"("DataIn"=w657, "FileName"=w649, "BG Time Taken (s)"=w658, "Save To File"=w669) -> ()  [unwired: 8 in]
              "BG Time (s)" <- w658
              "Backgate Display" <- w657
              "Computer Read Time (s)" <- w648
            }
            "Keithley 2450 Source" <- w637
          }
          frame "PostBackGateReset" {
            w687 = T11."Enabled" ("Disabled")
            n97 = call "SMU2450Init.vi"("Keithley Config"=w696, "error in (no error)"=w695, "Keithley 2400 Name"=w698) -> ("error out"=w694:errorcluster, "VISA resource name out"=w697:refnum<visa-resource-name>)  [unwired: 7 in]
            n98 = Enqueue Element(queue=w692, element="Read") -> ()  [unwired: 2 in, 3 out]
            n99 = property on="Backgate Display" class="XYGraph (strict)"("DisabledEnum"=w687) -> ()  [unwired: 2 in, 2 out]
            n100 = property on="Backgate" class="Bool"("DisabledEnum"=w687) -> ()  [unwired: 2 in, 2 out]
            n101 = local read "Aquire data"() -> (w686:bool)
            n102 = case shown="False" w686 {
              tunnel: w687 -> [w699 _]
              frame False {
                n103 = property on="File Name" class="Str"("DisabledEnum"=w699) -> ()  [unwired: 2 in, 2 out]
                n104 = property on="Save to File" class="Bool (strict)"("DisabledEnum"=w699) -> ()  [unwired: 2 in, 2 out]
              }
              frame True {
              }
            }
          }
          frame "Close" {
            # "Close and reinitialize keithley"
            n105 = call <instrlib>:"Close.vi"("error in (no error)"=w710, "VISA resource name"=w709) -> ("error out"=w708:errorcluster, "VISA resource name out"=w707:refnum<visa-resource-name>)  [unwired: 8 in]
            n106 = Flush Queue(queue=w705) -> (queue out=w706:refnum<queue>, error out=w704:errorcluster)  [unwired: 1 in, 1 out]
            n107 = call <instrlib>:"Close.vi"("error in (no error)"=w702, "VISA resource name"=w700) -> ("error out"=w701:errorcluster)  [unwired: 9 in]
            n108 = Enqueue Element(queue=w706, element="Initialize", error in (no error)=w704) -> ()  [unwired: 1 in, 3 out]
            n109 = Wait (ms)(milliseconds to wait=u32 100) -> ()  [unwired: 1 out]
          }
          frame "Exit" {
            # "Shut down Keithley loop"
            n110 = call <instrlib>:"Close.vi"("error in (no error)"=w715, "VISA resource name"=w717) -> ("error out"=w716:errorcluster)  [unwired: 8 in, 1 out]
            n111 = call <instrlib>:"Close.vi"("error in (no error)"=w713, "VISA resource name"=w714) -> ("error out"=w712:errorcluster)  [unwired: 9 in]
          }
        }
        "Keithley 2450 Sense" <- w521
        "DAQ 6510 Switch" <- w512
      }
      n112 = while "Timing" {
        tunnel: w61 -> [w82]
        shift-right: [w80] -> _
        shift-left: _ -> [w77]
        shift-right: [w79] -> _
        shift-left: _ -> [w78]
        shift-right: [w75] -> _
        shift-left: _ -> [w74]
        shift-right: [w73] -> _
        shift-left: _ -> [w72]
        tunnel: w60 -> [w71]
        stop <- w76 stop-if-true
        n113 = Dequeue Element(queue=w82) -> (queue out=w81:refnum<queue>, element=w70:string)  [unwired: 2 in, 2 out]
        n114 = case shown="\"EndTime\"" w70 {
          tunnel: w81 -> [w86 w107 w126 w143 w151 w155 w171 w192 w196 w200 w207 _]
          tunnel: [w84 w101 w121 w138 w146 w158 w172 w193 w197 _ w204 _] -> w80
          tunnel: [w91 w108 _ w140 w150 w159 w168 w180 w199 _ w205 _] -> w79
          tunnel: w78 -> [w85 _ _ w140 w150 w159 w168 _ w199 _ w205 _]
          tunnel: w77 -> [w84 _ w121 w138 w146 w158 w172 w193 w197 _ w204 _]
          tunnel: [_ _ _ _ _ _ _ _ _ _ _ TRUE] -> w76
          tunnel: [_ w106 w131 w139 w149 w160 w174 _ _ _ w202 _] -> w75
          tunnel: w74 -> [_ _ w130 w139 w149 w160 w174 _ _ _ w202 _]
          tunnel: [_ _ w127 w137 w148 w157 w173 _ w198 _ w203 _] -> w73
          tunnel: w72 -> [_ _ _ w137 w148 w157 w173 _ w198 _ w203 _]
          tunnel: w71 -> [_ w100 w125 _ _ _ _ w186 _ _ _ _]
          tunnel: [_ _ w123 w136 w144 w152 w169 _ w194 _ _ _] -> w68
          frame "Timeout", Default {
            # "Check the time vs endtime."
            n115 = Get Date/Time In Seconds() -> (seconds since 1Jan1904=w83:timestamp)
            n116 = Greater?(x=w83, y=w85) -> (0:w90:bool)
            n117 = Select(t="End" ("element"), s=w90, f="Timeout" ("element")) -> (s? t:f=w89:string)
            n118 = Enqueue Element(queue=w86, element=w89) -> ()  [unwired: 2 in, 3 out]
            n119 = property on="Aquire data" class="Bool (strict)"() -> ("Value"=w92:bool)  [unwired: 2 in, 2 out]
            n120 = case shown="False" w92 {
              tunnel: [w95 w98] -> w91
              tunnel: w85 -> [_ w98]
              frame False {
                n121 = Get Date/Time In Seconds() -> (seconds since 1Jan1904=w96:timestamp)
                n122 = To Quad Integer(1:w96) -> (0:w97:i64)
                n123 = Add(x=w97, y=i64 100) -> (x+y=w94:i64)
                n124 = To Time Stamp(1:w94) -> (0:w95:timestamp)
              }
              frame True {
              }
            }
            "Start Time" <- w84
          }
          frame "SetEnd" {
            # "If none script is selected, Set endtime, otherwise read script"
            n125 = property on="Script Contents" class="MCListbox (strict)"() -> ("ItemNames"=w106:string[][])  [unwired: 2 in, 2 out]
            n126 = call "HighlightRow.vi"("State"=enum16{"InitRows", "GetRows", "LastRow"}."InitRows", "Script Contents 2"=w100) -> ()  [unwired: 10 in]
            n127 = Get Date/Time In Seconds() -> (seconds since 1Jan1904=w101:timestamp)
            n128 = Array Size(array=w106) -> (size(s)=w105:i32[])
            n129 = Equal To 0?(x=w105) -> (x = 0?=w104:bool[])
            n130 = Index Array(array=w104) -> (element=w103:bool)  [unwired: 1 in]
            n131 = case shown="True" w103 {
              tunnel: [w109 w115] -> w108
              tunnel: ["PullAction" ("element") "Timeout" ("element")] -> w102
              tunnel: w101 -> [_ w116]
              frame False {
                n132 = Get Date/Time In Seconds() -> (seconds since 1Jan1904=w112:timestamp)
                n133 = To Quad Integer(1:w112) -> (0:w113:i64)
                n134 = Add(x=w113, y=i64 100) -> (x+y=w111:i64)
                n135 = To Time Stamp(1:w111) -> (0:w109:timestamp)
              }
              frame True {
                n136 = Multiply(x="Hours to Run", y=3600.0) -> (x*y=w118:dbl)
                n137 = Add(x=w118, y=w116) -> (x+y=w115:timestamp)
                "End Time" <- w115
              }
            }
            n138 = Enqueue Element(queue=w107, element=w102) -> ()  [unwired: 2 in, 3 out]
          }
          frame "PullAction" {
            # "Time, Control, Control Indicator, Value"
            n139 = call "HighlightRow.vi"("State"=enum16{"InitRows", "GetRows", "LastRow"}."GetRows", "Script Contents 2"=w125) -> ()  [unwired: 10 in]
            n140 = Delete From Array(array=w130, index (row)=0) -> (deleted portion=w127:string[], array with subset deleted=w131:string[][])  [unwired: 2 in]
            n141 = Index Array(array=w127, index=1) -> (element=w128:string)
            n142 = Enqueue Element(queue=w126, element=w128) -> ()  [unwired: 2 in, 3 out]
            n143 = Get Date/Time In Seconds() -> (seconds since 1Jan1904=w122:timestamp)
            n144 = Subtract(x=w122, y=w121) -> (x-y=w123:dbl)
          }
          frame "LED" {
            # "Change LED Values"
            n145 = control-ref of="Strobe"() -> (w134:refnum<vi>)
            n146 = control-ref of="Voltage (V)"() -> (w142:refnum<vi>)
            n147 = control-ref of="Duty Cycle"() -> (w133:refnum<vi>)
            n148 = control-ref of="Freq"() -> (w135:refnum<vi>)
            n149 = call "PushLED.vi"("Array"=w137, "Strobe"=w134, "Frequency"=w135, "Duty"=w133, "Voltage"=w142, "StartTime"=w138) -> ("Enqueue"=w141:string, "Current Time"=w136:dbl)  [unwired: 8 in]
            n150 = Enqueue Element(queue=w143, element=w141) -> ()  [unwired: 2 in, 3 out]
          }
          frame "Valves" {
            # "Change LED Values"
            n151 = control-ref of="Valves"() -> (w147:refnum<vi>)
            n152 = call "PushValves.vi"("StartTime"=w146, "Valves"=w147, "Array"=w148) -> ("Current Time"=w144:dbl, "Enqueue"=w145:string)  [unwired: 7 in]
            n153 = Enqueue Element(queue=w151, element=w145) -> ()  [unwired: 2 in, 3 out]
          }
          frame "MFC" {
            # "Change LED Values"
            n154 = control-ref of="MFC Set"() -> (w153:refnum<vi>)
            n155 = call "PushMFC.vi"("StartTime"=w158, "MFC Set 2"=w153, "Array"=w157) -> ("Current Time"=w152:dbl, "Boolean"=w154:bool, "Enqueue"=w156:string)  [unwired: 6 in]
            n156 = Enqueue Element(queue=w155, element=w156) -> ()  [unwired: 2 in, 3 out]
            n157 = case shown="True" w154 {
              frame False {
              }
              frame True {
                w163 = "MFC_IO" ("name (unnamed)")
                n158 = Obtain Queue(name (unnamed)=w163, element data type=w163) -> (queue out=w164:refnum<queue>)  [unwired: 3 in, 2 out]
                n159 = Enqueue Element(queue=w164, element="MFCSet") -> (queue out=w161:refnum<queue>)  [unwired: 2 in, 2 out]
                n160 = Release Queue(queue=w161) -> ()  [unwired: 2 in, 3 out]
              }
            }
          }
          frame "Backgate" {
            n161 = call "PushBackgate.vi"("StartTime"=w172, "Array"=w173) -> ("Current Time"=w169:dbl, "Backgate"=w165:bool, "Style"=w166:u16, "Enqueue"=w170:string, "Range (+-) (V)"=w167:dbl)  [unwired: 5 in]
            n162 = Enqueue Element(queue=w171, element=w170) -> ()  [unwired: 2 in, 3 out]
            n163 = case shown="True" w165 {
              tunnel: w167 -> [_ w176]
              tunnel: w166 -> [_ w175]
              frame False {
              }
              frame True {
                n164 = flat-sequence {
                  tunnel: w176 -> [w177]
                  tunnel: w175 -> [_]
                  frame #0 {
                    n165 = property on="Range (V)" class="DigNum (strict)"("Value"=w177) -> ()  [unwired: 2 in, 2 out]
                  }
                  frame #1 {
                    n166 = property on="DevBackgate" class="Bool (strict)"() -> ("Value"=w179:bool)  [unwired: 2 in, 2 out]
                    n167 = Not(x=w179) -> (.not. x?=w178:bool)
                    n168 = property on="DevBackgate" class="Bool (strict)"("Val(Sgnl)"=w178) -> ()  [unwired: 2 in, 2 out]
                  }
                }
              }
            }
          }
          frame "End" {
            # "End Script"
            n169 = call "HighlightRow.vi"("State"=enum16{"InitRows", "GetRows", "LastRow"}."LastRow", "Script Contents 2"=w186) -> ()  [unwired: 10 in]
            n170 = Enqueue Element(queue=w192, element="Timeout") -> ()  [unwired: 2 in, 3 out]
            n171 = property on="Timeout Stop" class="Bool (strict)"() -> ("Value"=w190:bool)  [unwired: 2 in, 2 out]
            n172 = Not(x=w190) -> (.not. x?=w189:bool)
            n173 = Get Date/Time In Seconds() -> (seconds since 1Jan1904=w183:timestamp)
            n174 = property on="Script Contents" class="MCListbox (strict)"("ColHdrString"=string[] [] ("Column Header Strings[]"), "ItemNames"=string[][] [] ("Item Names")) -> ()  [unwired: 2 in, 2 out]
            n175 = property on="Timeout Stop" class="Bool (strict)"("Val(Sgnl)"=w189) -> ()  [unwired: 2 in, 2 out]
            n176 = To Quad Integer(1:w183) -> (0:w184:i64)
            n177 = Add(x=w184, y=i64 100) -> (x+y=w182:i64)
            n178 = To Time Stamp(1:w182) -> (0:w180:timestamp)
          }
          frame "EndTime" {
            # "Wait for the endtime command"
            n179 = call "EndAction.vi"("StartTime"=w197, "Array"=w198) -> ("Current Time"=w194:dbl, "Enqueue"=w195:string)  [unwired: 8 in]
            n180 = Enqueue Element(queue=w196, element=w195) -> ()  [unwired: 2 in, 3 out]
          }
          frame "Close" {
            # "Flush shift registers"
            n181 = Enqueue Element(queue=w200, element="Timeout") -> ()  [unwired: 2 in, 3 out]
          }
          frame "Clear" {
            # "Clear the Multicollumn listbox"
            n182 = Enqueue Element(queue=w207, element="Timeout") -> ()  [unwired: 2 in, 3 out]
          }
          frame "Exit" {
            # "Exit the consumer loop"
          }
        }
        "Current Time (s)" <- w68
        n183 = Wait (ms)(milliseconds to wait=u32 50 ("millisecond multiple")) -> ()  [unwired: 1 out]
      }
      n184 = while {
        shift-right: [w436] -> _
        shift-left: _ -> [w439]
        shift-right: [w438] -> _
        shift-left: _ -> [w437]
        tunnel: w65 -> [w435]
        stop <- w440 stop-if-true
        n185 = Dequeue Element(queue=w435) -> (queue out=w442:refnum<queue>, element=w441:string)  [unwired: 2 in, 2 out]
        n186 = case shown="\"Strobe\"" w441 {
          tunnel: w442 -> [w450 w466 w479 w491 w499 _]
          tunnel: [_ _ _ _ _ TRUE] -> w440
          tunnel: [w447 w463 w475 w486 w496 w505] -> w436
          tunnel: w439 -> [_ w462 w476 w487 w494 w503]
          tunnel: [w448 w464 w477 w485 w497 w502] -> w438
          tunnel: w437 -> [_ w465 w477 w485 w498 w506]
          tunnel: "Freq" -> [_ w452 w478 w490 _ _]
          tunnel: 10.0 -> [w443 _ _ _ w493 w501]
          tunnel: [w443 w451 w470 w481 w493 w501] -> w432
          tunnel: "Duty Cycle" -> [_ _ w467 w483 _ _]
          frame "Initialize" {
            # "Initialize the DAQ"
            n187 = Enqueue Element(queue=w450, element="Send") -> ()  [unwired: 2 in, 3 out]
            n188 = call-poly <vilib>:"DAQmx Create Virtual Channel.vi"("physical channels"="AO_LED") -> ("task out"=w446:refnum<k21>, "error out"=w445:errorcluster)  [unwired: 13 in]
            n189 = call <vilib>:"DAQmx Start Task.vi"("task/channels in"=w446, "error in"=w445) -> ("task out"=w448:refnum<k21>, "error out"=w447:errorcluster)  [unwired: 12 in]
          }
          frame "Send", Default {
            # "Send data to the DAQ"
            n190 = local read "Strobe"() -> (w455:bool)
            n191 = Select(t="Strobe", s=w455, f="Send" ("element")) -> (s? t:f=w456:string)
            n192 = Select(t="Close" ("element"), s=w462, f=w456) -> (s? t:f=w460:string)
            n193 = call-poly <vilib>:"DAQmx Write.vi"("task/channels in"=w465, "data"="Voltage (V)", "error in"=w462) -> ("task out"=w464:refnum<k21>, "error out"=w463:errorcluster)  [unwired: 10 in, 1 out]
            n194 = Reciprocal(x=w452) -> (1/x=w454:dbl)
            n195 = Enqueue Element(queue=w466, element=w460) -> ()  [unwired: 2 in, 3 out]
            n196 = Multiply(x=1000.0, y=w454) -> (x*y=w451:dbl)
          }
          frame "Off" {
            n197 = call-poly <vilib>:"DAQmx Write.vi"("task/channels in"=w477, "data"=0.0 ("LED Voltage"), "error in"=w476) -> ("error out"=w475:errorcluster)  [unwired: 10 in, 2 out]
            n198 = Enqueue Element(queue=w479, element="Strobe") -> ()  [unwired: 2 in, 3 out]
            n199 = Reciprocal(x=w478) -> (1/x=w472:dbl)
            n200 = Multiply(x=w472, y=1000.0 ("x")) -> (x*y=w468:dbl)
            n201 = Subtract(x=1.0, y=w467) -> (x-y=w469:dbl)
            n202 = Multiply(x=w468, y=w469) -> (x*y=w470:dbl)
          }
          frame "Strobe" {
            (unwired) TRUE
            n203 = property on="Voltage (V)" class="Slide (strict)"() -> ("Value"=w488:dbl)  [unwired: 2 in, 2 out]
            n204 = call-poly <vilib>:"DAQmx Write.vi"("task/channels in"=w485, "data"=w488, "error in"=w487) -> ("error out"=w486:errorcluster)  [unwired: 10 in, 2 out]
            n205 = Enqueue Element(queue=w491, element="Off") -> ()  [unwired: 2 in, 3 out]
            n206 = Reciprocal(x=w490) -> (1/x=w489:dbl)
            n207 = Multiply(x=1000.0, y=w489) -> (x*y=w482:dbl)
            n208 = Multiply(x=w482, y=w483) -> (x*y=w481:dbl)
          }
          frame "Close" {
            (unwired) 50.0
            # "Close and reinit DAQ"
            n209 = call <vilib>:"DAQmx Stop Task.vi"("task/channels in"=w498, "error in"=w494) -> ("task out"=w497:refnum<k21>, "error out"=w495:errorcluster)  [unwired: 12 in]
            n210 = call <vilib>:"DAQmx Clear Task.vi"("task in"=w497, "error in"=w495) -> ("error out"=w496:errorcluster)  [unwired: 13 in]
            n211 = Enqueue Element(queue=w499, element="Initialize") -> ()  [unwired: 2 in, 3 out]
          }
          frame "Exit" {
            # "Shutdown DAQ"
            n212 = call <vilib>:"DAQmx Stop Task.vi"("task/channels in"=w506, "error in"=w503) -> ("task out"=w502:refnum<k21>, "error out"=w504:errorcluster)  [unwired: 12 in]
            n213 = call <vilib>:"DAQmx Clear Task.vi"("task in"=w502, "error in"=w504) -> ("error out"=w505:errorcluster)  [unwired: 13 in]
          }
        }
        "LED_AO" <- w436
        n214 = Wait (ms)(milliseconds to wait=w432) -> ()  [unwired: 1 out]
      }
      n215 = while {
        tunnel: w65 -> [w724]
        tunnel: w64 -> [w723]
        tunnel: w66 -> [w722]
        tunnel: w67 -> [w721]
        tunnel: w63 -> [w720]
        tunnel: w61 -> [w719]
        stop <- w725 stop-if-true
        n216 = event shown="[14] \"Strobe\": Value Change" {
          selector: _ -> [_ _ _ _ _ _ _ _ _ _ _ _ _ _ _ _ _ _ _]
          dyn-events: _ -> [_ _ _ _ _ _ _ _ _ _ _ _ _ _ _ _ _ _ _]
          timeout: _ -> [_ _ _ _ _ _ _ _ _ _ _ _ _ _ _ _ _ _ _]
          tunnel: [_ _ _ w740 _ _ _ _ _ _ _ _ _ _ _ _ _ _ _] -> w725
          tunnel: w724 -> [_ _ _ w741 _ _ _ _ _ w809 _ _ _ w876 w877 _ _ _ _]
          tunnel: w723 -> [_ _ _ w742 _ _ _ _ _ w810 _ _ _ _ _ _ _ _ _]
          tunnel: w722 -> [_ _ _ w743 _ w779 w783 _ _ w811 _ w850 w862 _ _ _ _ _ w912]
          tunnel: w721 -> [_ _ _ w744 _ _ _ w792 w793 w812 w838 _ _ _ _ _ _ _ _]
          tunnel: w720 -> [_ w726 _ w745 _ _ w781 _ _ w813 _ w849 w861 _ _ _ _ _ w913]
          tunnel: w719 -> [_ w728 _ w739 _ _ _ _ _ w802 _ _ _ _ _ _ _ _ _]
          event Timeout {
            n217 = event-data() -> ()  [unwired: 1 in, 1 out]
          }
          event "Aquire data": Value Change {
            n218 = event-data() -> ("NewVal"=w729:bool)  [unwired: 1 in]
            n219 = case shown="True" w729 {
              tunnel: w728 -> [_ w737]
              tunnel: "Aquire data" -> [_ w734]
              tunnel: w726 -> [_ w733]
              frame False {
              }
              frame True {
                w730 = T11."Disabled and Grayed Out" ("Disabled")
                n220 = Flush Queue(queue=w733) -> (queue out=w731:refnum<queue>)  [unwired: 1 in, 2 out]
                n221 = Flush Queue(queue=w737) -> (queue out=w736:refnum<queue>)  [unwired: 1 in, 2 out]
                n222 = Enqueue Element(queue=w736, element="SetEnd") -> ()  [unwired: 2 in, 3 out]
                n223 = Enqueue Element(queue=w731, element="ResetTimestamp") -> ()  [unwired: 2 in, 3 out]
                n224 = property on="Test Script" class="Ring (strict)"("DisabledEnum"=w730) -> ()  [unwired: 2 in, 2 out]
                n225 = property on="Aquire data" class="Bool (strict)"("DisabledEnum"=w730) -> ()  [unwired: 2 in, 2 out]
                n226 = property on="Aquire data 2" class="Bool (strict)"("DisabledEnum"=w730, "Value"=w734) -> ()  [unwired: 2 in, 2 out]
                n227 = property on="Save to File" class="Bool (strict)"("DisabledEnum"=w730) -> ()  [unwired: 2 in, 2 out]
                n228 = property on="File Name" class="Str"("DisabledEnum"=w730) -> ()  [unwired: 2 in, 2 out]
              }
            }
            n229 = property on="Plot Data" class="Bool (strict)"("Value"="Aquire data") -> ()  [unwired: 2 in, 2 out]
          }
          event "Aquire data 2": Value Change {
            n230 = event-data() -> ()  [unwired: 1 in, 6 out]
            n231 = property on="Aquire data" class="Bool (strict)"("Val(Sgnl)"="Aquire data 2") -> ()  [unwired: 2 in, 2 out]
          }
          event Panel Close? {
            n232 = event-data() -> ()  [unwired: 1 in, 1 out]
            n233 = Two Button Dialog(message="Are you sure you would like to close?", 2:"Yes" ("T button name (\"OK\")")) -> (T button?=w740:bool)  [unwired: 1 in]
            n234 = case shown="True" w740 {
              tunnel: w745 -> [_ w768]
              tunnel: w744 -> [_ w757]
              tunnel: w743 -> [_ w767]
              tunnel: w742 -> [_ w766]
              tunnel: w741 -> [_ w765]
              tunnel: w739 -> [_ w764]
              frame False {
              }
              frame True {
                w755 = "2200" ("name (unnamed)")
                w763 = "Exit" ("element")
                n235 = Flush Queue(queue=w757) -> (queue out=w756:refnum<queue>)  [unwired: 1 in, 2 out]
                n236 = Flush Queue(queue=w768) -> (queue out=w761:refnum<queue>)  [unwired: 1 in, 2 out]
                n237 = Flush Queue(queue=w767) -> (queue out=w760:refnum<queue>)  [unwired: 1 in, 2 out]
                n238 = Flush Queue(queue=w766) -> (queue out=w759:refnum<queue>)  [unwired: 1 in, 2 out]
                n239 = Flush Queue(queue=w764) -> (queue out=w762:refnum<queue>)  [unwired: 1 in, 2 out]
                n240 = Flush Queue(queue=w765) -> (queue out=w758:refnum<queue>)  [unwired: 1 in, 2 out]
                n241 = Enqueue Element At Opposite End(queue=w756, element=w763) -> ()  [unwired: 2 in, 3 out]
                n242 = Enqueue Element At Opposite End(queue=w760, element=w763) -> ()  [unwired: 2 in, 3 out]
                n243 = Enqueue Element At Opposite End(queue=w759, element=w763) -> ()  [unwired: 2 in, 3 out]
                n244 = Enqueue Element At Opposite End(queue=w758, element=w763) -> ()  [unwired: 2 in, 3 out]
                n245 = Enqueue Element At Opposite End(queue=w762, element=w763) -> ()  [unwired: 2 in, 3 out]
                n246 = Enqueue Element At Opposite End(queue=w761, element=w763) -> ()  [unwired: 2 in, 3 out]
                n247 = Obtain Queue(name (unnamed)=w755, element data type=w755) -> (queue out=w752:refnum<queue>, error out=w751:errorcluster)  [unwired: 3 in, 1 out]
                n248 = Flush Queue(queue=w752, error in (no error)=w751) -> (queue out=w749:refnum<queue>, error out=w750:errorcluster)  [unwired: 1 out]
                n249 = Enqueue Element(queue=w749, element="Exit", error in (no error)=w750) -> (queue out=w753:refnum<queue>)  [unwired: 1 in, 2 out]
                n250 = Release Queue(queue=w753) -> ()  [unwired: 2 in, 3 out]
              }
            }
            n251 = event-data("Discard?"=TRUE) -> ()  [unwired: 1 in, 1 out]
          }
          event "Backgate", "DevBackgate": Value Change {
            w769 = T11."Disabled and Grayed Out" ("Disabled")
            (unwired) FALSE ("StopBackgate")
            w775 = "Keithley" ("name (unnamed)")
            n252 = event-data() -> ()  [unwired: 1 in, 1 out]
            n253 = Obtain Queue(name (unnamed)=w775, element data type=w775) -> (queue out=w777:refnum<queue>, error out=w776:errorcluster)  [unwired: 3 in, 1 out]
            n254 = Flush Queue(queue=w777, error in (no error)=w776) -> (queue out=w774:refnum<queue>, error out=w773:errorcluster)  [unwired: 1 out]
            n255 = Enqueue Element(queue=w774, element="Backgate 2 2450", error in (no error)=w773) -> (queue out=w772:refnum<queue>, error out=w771:errorcluster)  [unwired: 1 in, 1 out]
            n256 = Release Queue(queue=w772, error in (no error)=w771) -> ()  [unwired: 1 in, 3 out]
            n257 = property on="Save to File" class="Bool (strict)"("DisabledEnum"=w769) -> ()  [unwired: 2 in, 2 out]
            n258 = property on="File Name" class="Str"("DisabledEnum"=w769) -> ()  [unwired: 2 in, 2 out]
            n259 = property on="Backgate" class="Bool"("DisabledEnum"=w769) -> ()  [unwired: 2 in, 2 out]
          }
          event "Clear DAQ": Value Change {
            n260 = event-data() -> ()  [unwired: 1 in, 1 out]
            n261 = Enqueue Element(queue=w779, element="Clear") -> ()  [unwired: 2 in, 3 out]
          }
          event Value Change {
            n262 = event-data() -> ()  [unwired: 1 in, 1 out]
            n263 = flat-sequence {
              tunnel: w783 -> [w787]
              tunnel: [w786] -> w782
              tunnel: w781 -> [w785]
              tunnel: [w784] -> w780
              tunnel: w782 -> [w790]
              tunnel: w780 -> [w789]
              frame #0 {
                n264 = Flush Queue(queue=w787) -> (queue out=w786:refnum<queue>)  [unwired: 1 in, 2 out]
                n265 = Flush Queue(queue=w785) -> (queue out=w784:refnum<queue>)  [unwired: 1 in, 2 out]
              }
              frame #1 {
                w788 = "Close" ("element")
                n266 = Enqueue Element(queue=w790, element=w788) -> ()  [unwired: 2 in, 3 out]
                n267 = Enqueue Element(queue=w789, element=w788) -> ()  [unwired: 2 in, 3 out]
              }
            }
          }
          event Value Change {
            n268 = event-data() -> ()  [unwired: 1 in, 6 out]
            n269 = Enqueue Element(queue=w792, element="tareFlow") -> ()  [unwired: 2 in, 3 out]
          }
          event Value Change {
            n270 = event-data() -> ()  [unwired: 1 in, 1 out]
            n271 = Enqueue Element(queue=w793, element="tareAbsP") -> ()  [unwired: 2 in, 3 out]
          }
          event "Stop", "Timeout Stop": Value Change {
            (unwired) TRUE ("StopBackgate")
            w796 = "2200" ("name (unnamed)")
            w795 = T11."Enabled" ("Disabled")
            # "Make string writeable"
            n272 = event-data() -> ()  [unwired: 1 in, 1 out]
            n273 = flat-sequence {
              tunnel: w809 -> [w817]
              tunnel: w810 -> [w819]
              tunnel: w811 -> [w821]
              tunnel: w812 -> [w823]
              tunnel: w813 -> [w825]
              tunnel: [w824] -> w808
              tunnel: [w822] -> w807
              tunnel: [w820] -> w806
              tunnel: [w818] -> w805
              tunnel: [w816] -> w804
              tunnel: w802 -> [w815]
              tunnel: [w814] -> w803
              tunnel: w808 -> [w833]
              tunnel: w807 -> [w829]
              tunnel: w806 -> [w830]
              tunnel: w805 -> [w831]
              tunnel: w804 -> [w832]
              tunnel: w803 -> [w828]
              frame #0 {
                n274 = Flush Queue(queue=w815) -> (queue out=w814:refnum<queue>)  [unwired: 1 in, 2 out]
                n275 = Flush Queue(queue=w825) -> (queue out=w824:refnum<queue>)  [unwired: 1 in, 2 out]
                n276 = Flush Queue(queue=w823) -> (queue out=w822:refnum<queue>)  [unwired: 1 in, 2 out]
                n277 = Flush Queue(queue=w821) -> (queue out=w820:refnum<queue>)  [unwired: 1 in, 2 out]
                n278 = Flush Queue(queue=w819) -> (queue out=w818:refnum<queue>)  [unwired: 1 in, 2 out]
                n279 = Flush Queue(queue=w817) -> (queue out=w816:refnum<queue>)  [unwired: 1 in, 2 out]
              }
              frame #1 {
                w827 = "Close" ("element")
                n280 = Enqueue Element At Opposite End(queue=w829, element=w827) -> ()  [unwired: 2 in, 3 out]
                n281 = Enqueue Element At Opposite End(queue=w830, element=w827) -> ()  [unwired: 2 in, 3 out]
                n282 = Enqueue Element At Opposite End(queue=w831, element=w827) -> ()  [unwired: 2 in, 3 out]
                n283 = Enqueue Element At Opposite End(queue=w832, element=w827) -> ()  [unwired: 2 in, 3 out]
                n284 = Enqueue Element At Opposite End(queue=w828, element="Clear") -> ()  [unwired: 2 in, 3 out]
                n285 = Enqueue Element At Opposite End(queue=w833, element=w827) -> ()  [unwired: 2 in, 3 out]
              }
              frame #2 {
                n286 = invoke on="Aquire data 2" class="Bool (strict)" method="Reinit To Default"() -> ()  [unwired: 3 in, 3 out]
                n287 = invoke on="Test Script" class="Ring (strict)" method="Reinit To Default"() -> ()  [unwired: 3 in, 3 out]
                n288 = invoke on="File Name" class="Str" method="Reinit To Default"() -> ()  [unwired: 3 in, 3 out]
                n289 = invoke on="Save to File" class="Bool (strict)" method="Reinit To Default"() -> ()  [unwired: 3 in, 3 out]
                n290 = invoke on="Aquire data" class="Bool (strict)" method="Reinit To Default"() -> ()  [unwired: 3 in, 3 out]
              }
              frame #3 {
                n291 = property on="Test Script" class="Ring (strict)"() -> ("Strings []"=w834:string[])  [unwired: 2 in, 2 out]
                n292 = Search 1D Array(1D array=w834, element="None") -> (index of element=w835:i32)  [unwired: 1 in]
                n293 = property on="Test Script" class="Ring (strict)"("Val(Sgnl)"=w835) -> ()  [unwired: 2 in, 2 out]
              }
            }
            n294 = property on="Plot Data" class="Bool (strict)"("Value"=FALSE ("Plot Data")) -> ()  [unwired: 2 in, 2 out]
            n295 = property on="File Name" class="Str"("DisabledEnum"=w795) -> ()  [unwired: 2 in, 2 out]
            n296 = property on="Aquire data 2" class="Bool (strict)"("DisabledEnum"=w795) -> ()  [unwired: 2 in, 2 out]
            n297 = property on="Aquire data" class="Bool (strict)"("DisabledEnum"=w795) -> ()  [unwired: 2 in, 2 out]
            n298 = property on="Save to File" class="Bool (strict)"("DisabledEnum"=w795) -> ()  [unwired: 2 in, 2 out]
            n299 = property on="Test Script" class="Ring (strict)"("DisabledEnum"=w795) -> ()  [unwired: 2 in, 2 out]
            n300 = property on="Backgate" class="Bool"("DisabledEnum"=w795) -> ()  [unwired: 2 in, 2 out]
            n301 = Obtain Queue(name (unnamed)=w796, element data type=w796) -> (queue out=w798:refnum<queue>)  [unwired: 3 in, 2 out]
            n302 = Flush Queue(queue=w798) -> (queue out=w799:refnum<queue>)  [unwired: 1 in, 2 out]
            n303 = Enqueue Element(queue=w799, element="Close") -> (queue out=w800:refnum<queue>)  [unwired: 2 in, 2 out]
            n304 = Release Queue(queue=w800) -> ()  [unwired: 2 in, 3 out]
          }
          event "MFC Set": Value Change {
            n305 = event-data() -> ("OldVal"=w839:T6[], "NewVal"=w837:T6[])  [unwired: 1 in]
            n306 = for {
              tunnel: w839 -> [w845] mode=indexing
              tunnel: w838 -> [w841]
              tunnel: w837 -> [w840] mode=indexing
              i -> [w843]
              stop <- w842 stop-if-true
              n307 = Not Equal?(x=w845, y=w840) -> (x != y?=w844:T13)
              n308 = Unbundle(w844) -> ("set 1"=w842:bool)  [unwired: 1 out]
              n309 = case shown="True" w842 {
                tunnel: w841 -> [_ w846]
                frame False {
                }
                frame True {
                  n310 = Enqueue Element(queue=w846, element="MFCSet") -> ()  [unwired: 2 in, 3 out]
                }
              }
              "MFC Index" <- w843
            }
          }
          event "File Name": Value Change {
            n311 = event-data() -> ()  [unwired: 1 in, 1 out]
            n312 = flat-sequence {
              tunnel: w850 -> [w855]
              tunnel: [w854] -> w851
              tunnel: w849 -> [w853]
              tunnel: [w852] -> w848
              tunnel: w851 -> [w858]
              tunnel: w848 -> [w857]
              frame #0 {
                n313 = Flush Queue(queue=w855) -> (queue out=w854:refnum<queue>)  [unwired: 1 in, 2 out]
                n314 = Flush Queue(queue=w853) -> (queue out=w852:refnum<queue>)  [unwired: 1 in, 2 out]
              }
              frame #1 {
                w856 = "Close" ("element")
                n315 = Enqueue Element(queue=w858, element=w856) -> ()  [unwired: 2 in, 3 out]
                n316 = Enqueue Element(queue=w857, element=w856) -> ()  [unwired: 2 in, 3 out]
              }
            }
          }
          event "Save to File": Value Change {
            n317 = event-data() -> ("NewVal"=w864:bool)  [unwired: 1 in]
            n318 = flat-sequence {
              tunnel: w862 -> [w868]
              tunnel: [w867] -> w863
              tunnel: w861 -> [w866]
              tunnel: [w865] -> w860
              tunnel: w863 -> [w871]
              tunnel: w860 -> [w870]
              frame #0 {
                n319 = Flush Queue(queue=w868) -> (queue out=w867:refnum<queue>)  [unwired: 1 in, 2 out]
                n320 = Flush Queue(queue=w866) -> (queue out=w865:refnum<queue>)  [unwired: 1 in, 2 out]
              }
              frame #1 {
                w869 = "Close" ("element")
                n321 = Enqueue Element(queue=w870, element=w869) -> ()  [unwired: 2 in, 3 out]
                n322 = Enqueue Element(queue=w871, element=w869) -> ()  [unwired: 2 in, 3 out]
              }
            }
            n323 = case shown="False" w864 {
              tunnel: [T11."Enabled" ("Disabled") T11."Disabled and Grayed Out" ("Disabled")] -> w859
              frame False {
              }
              frame True {
              }
            }
            n324 = property on="File Name" class="Str"("DisabledEnum"=w859) -> ()  [unwired: 2 in, 2 out]
          }
          event "Voltage (V)": Value Change {
            n325 = event-data() -> ()  [unwired: 1 in, 1 out]
            n326 = Enqueue Element(queue=w876, element="Send") -> ()  [unwired: 2 in, 3 out]
            n327 = property on="Strobe" class="Bool (strict)"("Val(Sgnl)"=FALSE ("Value (Signaling)")) -> ()  [unwired: 2 in, 2 out]
          }
          event "Strobe": Value Change {
            n328 = event-data() -> ("NewVal"=w878:bool)  [unwired: 1 in]
            n329 = case shown="True" w878 {
              tunnel: w877 -> [w880 w882]
              frame False {
                n330 = Flush Queue(queue=w880) -> (queue out=w879:refnum<queue>)  [unwired: 1 in, 2 out]
                n331 = Enqueue Element(queue=w879, element="Send") -> ()  [unwired: 2 in, 3 out]
              }
              frame True {
                n332 = Flush Queue(queue=w882) -> (queue out=w883:refnum<queue>)  [unwired: 1 in, 2 out]
                n333 = Enqueue Element(queue=w883, element="Strobe") -> ()  [unwired: 2 in, 3 out]
              }
            }
          }
          event "Test Script": Mouse Enter {
            n334 = event-data() -> ("CtlRef"=w890:refnum<vi>)  [unwired: 1 in]
            n335 = property class="Ring (strict)"(reference=w890) -> ("Strings []"=w889:string[], "Value"=w888:u16)  [unwired: 1 in, 2 out]
            n336 = Index Array(array=w889, index=w888) -> (element=w887:string)
            n337 = call "PopulateRing.vi"() -> ("Array"=w886:string[])  [unwired: 10 in, 1 out]
            n338 = Search 1D Array(1D array=w886, element=w887) -> (index of element=w885:i32)  [unwired: 1 in]
            n339 = property on="Test Script" class="Ring (strict)"("Strings []"=w886, "Value"=w885) -> ()  [unwired: 2 in, 2 out]
          }
          event "Test Script": Value Change {
            n340 = event-data() -> ("NewVal"=w897:u16)  [unwired: 1 in]
            n341 = property on="Test Script" class="Ring (strict)"() -> ("Strings []"=w896:string[])  [unwired: 2 in, 2 out]
            n342 = Index Array(array=w896, index=w897) -> (element=w895:string)
            n343 = call "ReadScript.vi"("String"=w895) -> ("all rows"=w894:string[][])  [unwired: 9 in, 1 out]
            n344 = Delete From Array(array=w894, index (row)=0) -> (deleted portion=w891:string[], array with subset deleted=w893:string[][])  [unwired: 2 in]
            n345 = property on="Script Contents" class="MCListbox (strict)"("ItemNames"=w893, "ColHdrString"=w891) -> ()  [unwired: 2 in, 2 out]
          }
          event "# of Sensors": Value Change {
            n346 = event-data() -> ("NewVal"=w899:dbl)  [unwired: 1 in, 5 out]
            n347 = Decrement(x=w899) -> (x-1=w903:dbl)
            n348 = Array Subset(array=string[] ["Resistance 2", "Resistance 3", "Resistance 4", "Resistance 5", "Resistance 6", "Resistance 7", "Resistance 8", "Resistance 9"], length=w903) -> (w906:string[])  [unwired: 1 in]
            n349 = Insert Into Array(array="Names default", new element=w906) -> (→"Names":string[])  [unwired: 1 in]
            n350 = for {
              N: 9 -> [_]
              tunnel: [w908] -> w900 mode=indexing
              tunnel: w899 -> [w910]
              i -> [w909]
              n351 = Greater?(x=w910, y=w909) -> (0:w908:bool)
            }
            n352 = Add(x=w899, y=5.0) -> (x+y=w901:dbl)
            n353 = property on="CvsV" class="XYGraph (strict)"("LegNumRows"=w899) -> ()  [unwired: 2 in, 2 out]
            n354 = property on="Waveform Chart" class="WFChart (strict)"("LegNumRows"=w901) -> ()  [unwired: 2 in, 2 out]
            n355 = property on="Sensors" class="Arr (strict)"("Value"=w900) -> ()  [unwired: 2 in, 2 out]
          }
          event Value Change {
            n356 = event-data() -> ()  [unwired: 1 in, 1 out]
            n357 = flat-sequence {
              tunnel: w913 -> [w918]
              tunnel: [w917] -> w914
              tunnel: w912 -> [w916]
              tunnel: [w915] -> w911
              tunnel: w914 -> [w921]
              tunnel: w911 -> [w920]
              frame #0 {
                n358 = Flush Queue(queue=w918) -> (queue out=w917:refnum<queue>)  [unwired: 1 in, 2 out]
                n359 = Flush Queue(queue=w916) -> (queue out=w915:refnum<queue>)  [unwired: 1 in, 2 out]
              }
              frame #1 {
                w919 = "Close" ("element")
                n360 = Enqueue Element(queue=w920, element=w919) -> ()  [unwired: 2 in, 3 out]
                n361 = Enqueue Element(queue=w921, element=w919) -> ()  [unwired: 2 in, 3 out]
              }
            }
          }
        }
      }
      n362 = while {
        shift-right: [w212] -> _
        shift-left: _ -> [w215]
        shift-right: [w214] -> _
        shift-left: _ -> [w213]
        tunnel: w67 -> [w211]
        stop <- w216 stop-if-true
        n363 = Dequeue Element(queue=w211) -> (queue out=w218:refnum<queue>, element=w217:string)  [unwired: 2 in, 2 out]
        n364 = case shown="\"queryFormat\", Default" w217 {
          tunnel: w218 -> [w228 w237 w246 w256 _ w276 _]
          tunnel: [_ _ _ _ _ _ TRUE] -> w216
          tunnel: [w221 w230 w251 w258 w269 w272 w282] -> w212
          tunnel: w215 -> [_ w240 w244 w259 w270 w274 w280]
          tunnel: [w220 w235 w247 w254 w267 w271 w278] -> w214
          tunnel: w213 -> [_ w239 w248 w255 w268 w275 w279]
          tunnel: "MFC Config" -> [w226 w234 w250 w257 _ _ _]
          frame "Initialize" {
            # "Initialize the Visa COM."
            n365 = Unbundle By Name(w226) -> ("MFC COM Port"=w225:refnum<visa-resource-name>, "baud rate (9600)"=w224:u32)
            n366 = Enqueue Element(queue=w228, element="queryFormat") -> ()  [unwired: 2 in, 3 out]
            n367 = call-poly "VISA Configure Serial Port"("VISA resource name"=w225, "termination char\n(0xA = '\\n' = LF)"=u8 13 ("termination char\n(0xA = '\\n' = LF)"), "Enable Termination\nChar (T)"=TRUE ("Enable Termination\nChar (T)"), "baud rate (9600)"=w224) -> ("VISA resource name out"=w227:refnum<visa-resource-name>, "error out"=w219:errorcluster)  [unwired: 10 in]
            n368 = VISA Clear(VISA resource name=w227, error in (no error)=w219) -> (VISA resource name out=w220:refnum<visa-resource-name>, error out=w221:errorcluster)
          }
          frame "queryFormat", Default {
            n369 = Unbundle By Name(w234) -> ("Device ID's"=w238:string[])
            n370 = Select(t="Close" ("element"), s=w240, f="queryFormat" ("element")) -> (s? t:f=w236:string)
            n371 = Enqueue Element(queue=w237, element=w236) -> ()  [unwired: 2 in, 3 out]
            n372 = call "MFCquery.vi"("error in (no error)"=w240, "Device ID's"=w238, "VISA Refnum in"=w239) -> ("error out"=w231:errorcluster, "Array"=w233:string[], "VISA Refnum out"=w235:refnum<visa-resource-name>)  [unwired: 6 in]
            n373 = call "MFCstringFormat.vi"("error in (no error)"=w231, "Array"=w233) -> ("error out"=w230:errorcluster, "Array Out"=→"MFCArray":T7[])  [unwired: 7 in]
          }
          frame "tareFlow" {
            n374 = Unbundle By Name(w250) -> ("Device ID's"=w249:string[])
            n375 = Select(t="Close" ("element"), s=w244, f="queryFormat" ("element")) -> (s? t:f=w253:string)
            n376 = Enqueue Element(queue=w246, element=w253) -> ()  [unwired: 2 in, 3 out]
            n377 = call "MFCCMD.vi"("error in (no error)"=w244, "cmd"="v", "Device ID's"=w249, "VISA Refnum in"=w248) -> ("error out"=w251:errorcluster, "VISA Refnum out"=w247:refnum<visa-resource-name>)  [unwired: 6 in]
          }
          frame "tareAbsP" {
            n378 = Unbundle By Name(w257) -> ("Device ID's"=w263:string[])
            n379 = Select(t="Close" ("element"), s=w259, f="queryFormat" ("element")) -> (s? t:f=w264:string)
            n380 = Enqueue Element(queue=w256, element=w264) -> ()  [unwired: 2 in, 3 out]
            n381 = call "MFCCMD.vi"("error in (no error)"=w259, "cmd"="pc", "Device ID's"=w263, "VISA Refnum in"=w255) -> ("error out"=w258:errorcluster, "VISA Refnum out"=w254:refnum<visa-resource-name>)  [unwired: 6 in]
          }
          frame "MFCSet" {
            # "Push the MFC values."
            n382 = local read "MFC Index"() -> (w266:i32)
            n383 = call "MFC_Setpoint.vi"("error in"=w270, "index"=w266, "MFC Set"="MFC Set", "VISA Refnum in"=w268) -> ("error out"=w269:errorcluster, "VISA Refnum out"=w267:refnum<visa-resource-name>)  [unwired: 6 in]
          }
          frame "Close" {
            # "Close and reinitialize the Visa"
            n384 = VISA Clear(VISA resource name=w275, error in (no error)=w274) -> (VISA resource name out=w271:refnum<visa-resource-name>, error out=w273:errorcluster)
            n385 = VISA Close(VISA resource name=w271, error in (no error)=w273) -> (error out=w272:errorcluster)
            n386 = Enqueue Element(queue=w276, element="Initialize") -> ()  [unwired: 2 in, 3 out]
          }
          frame "Exit" {
            # "Shut down Visa."
            n387 = VISA Clear(VISA resource name=w279, error in (no error)=w280) -> (VISA resource name out=w278:refnum<visa-resource-name>, error out=w281:errorcluster)
            n388 = VISA Close(VISA resource name=w278, error in (no error)=w281) -> (error out=w282:errorcluster)
          }
        }
        "MFC_IO" <- w212
        n389 = Wait (ms)(milliseconds to wait=u32 100 ("millisecond multiple")) -> ()  [unwired: 1 out]
      }
      n390 = while {
        shift-right: [w331] -> _
        shift-left: _ -> [w334]
        shift-right: [w333] -> _
        shift-left: _ -> [w332]
        shift-right: [w330] -> _
        shift-left: _ -> [w328]
        tunnel: w66 -> [w329]
        shift-right: [w324] -> _
        shift-left: _ -> [w323]
        stop <- w326 stop-if-true
        n391 = Dequeue Element(queue=w329, timeout in ms (-1)=50) -> (queue out=w336:refnum<queue>, element=w335:string)  [unwired: 1 in, 2 out]
        n392 = case shown="\"Read\", Default" w335 {
          tunnel: w336 -> [w338 _ w372 w406 _ w420 _]
          tunnel: [_ _ _ _ _ _ TRUE] -> w326
          tunnel: [w342 w356 w367 w398 w416 w418 w428] -> w331
          tunnel: w334 -> [_ w356 w369 w404 w414 w419 w425]
          tunnel: [w347 w357 w375 w382 w417 _ _] -> w333
          tunnel: w332 -> [_ w357 w377 w382 w417 w421 w429]
          tunnel: [dbl[] [] _ w368 _ dbl[] [] _ _] -> w330
          tunnel: w328 -> [_ _ _ w396 _ _ _]
          tunnel: "DAQ Config" -> [w345 _ w365 w393 _ _ _]
          tunnel: [_ w355 w364 w390 w412 _ _] -> w324
          tunnel: w323 -> [_ _ w364 w388 w412 _ _]
          frame "Initialize" {
            w350 = 10123 items=["Finite Samples"=10178, "Continuous Samples"=10123, "Hardware Timed Single Point"=12522] ("sample mode")
            w343 = 10083 items=["default"=-1, "RSE"=10083, "NRSE"=10078, "Differential"=10106, "Pseudodifferential"=12529] ("input terminal configuration")
            # "Initialize the DAQ with given settings."
            n393 = Unbundle By Name(w345) -> ("Samples/Channel/s"=w344:dbl)
            n394 = Select(t="File" ("element"), s="Save to File", f="Read") -> (s? t:f=w337:string)
            n395 = Enqueue Element(queue=w338, element=w337) -> ()  [unwired: 2 in, 3 out]
            n396 = call-poly <vilib>:"DAQmx Create Virtual Channel.vi"("maximum value"=5.0, "minimum value"=0.0, "input terminal configuration"=w343, "physical channels"="DAQ channels") -> ("task out"=w351:refnum<k21>, "error out"=w352:errorcluster)  [unwired: 10 in]
            n397 = call-poly <vilib>:"DAQmx Timing.vi"("task/channels in"=w351, "sample mode"=w350, "rate"=w344, "error in"=w352) -> ("task out"=w347:refnum<k21>, "error out"=w353:errorcluster)  [unwired: 10 in]
            n398 = call <vilib>:"DAQmx Start Task.vi"("task/channels in"=w347, "error in"=w353) -> ("error out"=w342:errorcluster)  [unwired: 12 in, 1 out]
          }
          frame "File" {
            # "If no error, create a path for the file saving."
            n399 = case shown="No Error" w356 {
              tunnel: [w359 _] -> w355
              frame No Error {
                w358 = u16 1 items=["Check", "Init"] ("Ring")
                n400 = call "OpenFileDAQ.vi"("DAQ File Name"="File Name") -> ("appended path"=w359:path)  [unwired: 7 in, 2 out]
                n401 = call "Tnaught.vi"("Ring"=w358) -> ()  [unwired: 10 in, 1 out]
              }
              frame Error {
              }
            }
          }
          frame "Read", Default {
            # "Read and mean the DAQ data to provide accurate result.  Update unprocessed samples"
            n402 = Unbundle By Name(w365) -> ("Samples to Average"=w374:dbl)
            n403 = property class="DAQmx Read"(reference=w377, error in=w369) -> (reference out=w376:refnum<k21>, error out=w373:errorcluster, "AvailSampPerChan"=→"Unprocessed Samples in Queue":u32)
            n404 = Select(t="Close" ("element"), s=w369, f="Process" ("element")) -> (s? t:f=w378:string)
            n405 = call-poly <vilib>:"DAQmx Read.vi"("task/channels in"=w376, "number of samples per channel"=w374, "error in"=w373) -> ("task out"=w375:refnum<k21>, "data"=w363:waveform(dbl)[], "error out"=w367:errorcluster)  [unwired: 10 in]
            n406 = Enqueue Element(queue=w372, element=w378) -> ()  [unwired: 2 in, 3 out]
            n407 = for {
              tunnel: w363 -> [w379] mode=indexing
              tunnel: [w380] -> w368 mode=indexing
              n408 = call-poly <vilib>:"Mean.vi"("X"=w379) -> ("mean"=w380:dbl)  [unwired: 1 out]
            }
            n409 = Index Array(array=w363) -> (element=w362:waveform(dbl))  [unwired: 1 in]
            n410 = Unbundle By Name(w362) -> ("t0"=→"t0":timestamp)
          }
          frame "Process" {
            # "Process the data and plot/save to file (maybe).  Update the indicators."
            n411 = local read "Resistance Proper"() -> (w381:dbl[][])
            n412 = local read "MFCArray"() -> (w386:T7[])
            n413 = call "conversionsTempEth.vi"("Array"=w396, "error in (no error)"=w404, "Parameters"=w393) -> ("error out"=w403:errorcluster, "T"=w400:dbl, "RH"=w401:dbl, "Ethanol"=w402:dbl)  [unwired: 5 in]
            "Eth" <- w402
            "RH" <- w401
            "T" <- w400
            n414 = Select(t="Close" ("element"), s=w404, f="Read") -> (s? t:f=w405:string)
            n415 = call "Graph.vi"("Resistances In"=w381, "Array in"=w386, "error in (no error)"=w403, "T  (ºC)"=w400, "RH  (%)"=w401, "Ethanol (%)"=w402) -> ("error out"=w399:errorcluster, "Cluster"=w397:T14)  [unwired: 4 in]
            n416 = Enqueue Element(queue=w406, element=w405) -> ()  [unwired: 2 in, 3 out]
            n417 = local read "t0"() -> (w387:timestamp)
            n418 = call "waveformTimeKeep.vi"("t0"=w387, "DAQ Settings"=w393, "error in (no error)"=w399, "Cluster"=w397) -> ("error out"=w398:errorcluster, "Samples/second"=→"DPS":dbl, "appended array"=w385:waveform(dbl)[])  [unwired: 5 in]
            n419 = Get Date/Time In Seconds() -> (seconds since 1Jan1904=w383:timestamp)
            n420 = local read "Aquire data"() -> (w391:bool)
            n421 = for {
              tunnel: [w408] -> w384 mode=indexing
              tunnel: w385 -> [w410] mode=indexing
              tunnel: w383 -> [w409]
              n422 = Bundle By Name(cluster=w410, "t0"=w409) -> (w408:waveform(dbl))
            }
            n423 = local read "Names"() -> (w389:string[])
            n424 = call "DAQFileIO.vi"("Aquire Data"=w391, "File Path In"=w388, "Names"=w389, "data"=w385) -> ("file path out"=w390:path)  [unwired: 6 in, 1 out]
            n425 = case shown="True" "Plot Data" {
              tunnel: w384 -> [_ w411]
              frame False {
              }
              frame True {
                "Waveform Chart" <- w411
              }
            }
          }
          frame "Clear" {
            # "Clear the DAQ waveform chart."
            n426 = property on="Waveform Chart" class="WFChart (strict)"(error in=w414, "History Data"=waveform(dbl)[][] []) -> (error out=w416:errorcluster)  [unwired: 1 in, 1 out]
          }
          frame "Close" {
            # "Close and Reinitialize the DAQ."
            n427 = call <vilib>:"DAQmx Stop Task.vi"("task/channels in"=w421, "error in"=w419) -> ("task out"=w422:refnum<k21>, "error out"=w423:errorcluster)  [unwired: 12 in]
            n428 = Enqueue Element(queue=w420, element="Initialize") -> ()  [unwired: 2 in, 3 out]
            n429 = call <vilib>:"DAQmx Clear Task.vi"("task in"=w422, "error in"=w423) -> ("error out"=w418:errorcluster)  [unwired: 13 in]
          }
          frame "Exit" {
            # "Shut down the DAQ."
            n430 = call <vilib>:"DAQmx Stop Task.vi"("task/channels in"=w429, "error in"=w425) -> ("task out"=w426:refnum<k21>, "error out"=w427:errorcluster)  [unwired: 12 in]
            n431 = call <vilib>:"DAQmx Clear Task.vi"("task in"=w426, "error in"=w427) -> ("error out"=w428:errorcluster)  [unwired: 13 in]
          }
        }
        "DAQ_IO (RH,Temp,Eth)" <- w331
      }
      n432 = while {
        shift-right: [w286] -> _
        shift-left: _ -> [w289]
        shift-right: [w288] -> _
        shift-left: _ -> [w287]
        tunnel: w64 -> [w285]
        stop <- w290 stop-if-true
        n433 = Dequeue Element(queue=w285) -> (queue out=w292:refnum<queue>, element=w291:string)  [unwired: 2 in, 2 out]
        n434 = case shown="\"Send\", Default" w291 {
          tunnel: w292 -> [w300 w309 w315 _]
          tunnel: [_ _ _ TRUE] -> w290
          tunnel: [w297 w306 w310 w319] -> w286
          tunnel: w289 -> [_ w305 w311 w317]
          tunnel: [w298 w307 w313 w320] -> w288
          tunnel: w287 -> [_ w308 w314 w321]
          frame "Initialize" {
            w294 = 0 items=["one channel for each line", "one channel for all lines"] ("line grouping")
            # "Initialize the DAQ"
            n435 = call-poly <vilib>:"DAQmx Create Virtual Channel.vi"("lines"="DO_Valves", "line grouping"=w294) -> ("task out"=w296:refnum<k21>, "error out"=w295:errorcluster)  [unwired: 12 in]
            n436 = Enqueue Element(queue=w300, element="Send") -> ()  [unwired: 2 in, 3 out]
            n437 = call <vilib>:"DAQmx Start Task.vi"("task/channels in"=w296, "error in"=w295) -> ("task out"=w298:refnum<k21>, "error out"=w297:errorcluster)  [unwired: 12 in]
          }
          frame "Send", Default {
            # "Send Valve data"
            n438 = Select(t="Close" ("element"), s=w305, f="Send" ("element")) -> (s? t:f=w302:string)
            n439 = Enqueue Element(queue=w309, element=w302) -> ()  [unwired: 2 in, 3 out]
            n440 = call-poly <vilib>:"DAQmx Write.vi"("task/channels in"=w308, "data"="Valves", "error in"=w305) -> ("task out"=w307:refnum<k21>, "error out"=w306:errorcluster)  [unwired: 10 in, 1 out]
          }
          frame "Close" {
            # "Close and reinit the DAQ"
            n441 = call <vilib>:"DAQmx Stop Task.vi"("task/channels in"=w314, "error in"=w311) -> ("task out"=w313:refnum<k21>, "error out"=w312:errorcluster)  [unwired: 12 in]
            n442 = call <vilib>:"DAQmx Clear Task.vi"("task in"=w313, "error in"=w312) -> ("error out"=w310:errorcluster)  [unwired: 13 in]
            n443 = Enqueue Element(queue=w315, element="Initialize") -> ()  [unwired: 2 in, 3 out]
          }
          frame "Exit" {
            # "Shut down the DAQ"
            n444 = call <vilib>:"DAQmx Stop Task.vi"("task/channels in"=w321, "error in"=w317) -> ("task out"=w320:refnum<k21>, "error out"=w318:errorcluster)  [unwired: 12 in]
            n445 = call <vilib>:"DAQmx Clear Task.vi"("task in"=w320, "error in"=w318) -> ("error out"=w319:errorcluster)  [unwired: 13 in]
          }
        }
        "3-Valve_DO" <- w286
        n446 = Wait (ms)(milliseconds to wait=u32 50) -> ()  [unwired: 1 out]
      }
    }
    frame #2 {
      # "In development environment, do not close the panel"
      n447 = property class="App"() -> ("App.Kind"=w923:T8)  [unwired: 2 in, 2 out]
      n448 = Equal?(x=w923, y=T8."Run Time System" ("Application:Kind")) -> (x = y?=w924:bool)
      n449 = case shown="False" w924 {
        frame False {
        }
        frame True {
          n450 = Quit LabVIEW() -> ()  [unwired: 1 in]
        }
      }
    }
  }
